vi "Auto.vi"() -> ()   [LabVIEW 2017]
uses:
  Control/Saurabh/prosucer_consumer_enum.ctl
  <vilib>/Utility/error.llb/DialogType.ctl
  <vilib>/Utility/file.llb/Read Delimited Spreadsheet (string).vi
  Global/Global 1.vi
  Global/DATA LOG.vi
  <userlib>/_OpenG.lib/comparison/comparison.llb/String Changed__ogtk.vi
  <vilib>/addons/database/Connection.llb/DB Tools Open Connec (String).vi
  <vilib>/addons/database/NI_Database_API.lvlib
  <vilib>/regexp/Match Regular Expression.xnode
panel:
  out "LOG DATA":string
  out "scanner value":string
  out "PRIVIOUS DATA":string
  out "array w/ subset deleted":dbl[](array[numeric])
  out "LOG DATA 2":dbl[](array[numeric])
  out "DATA":bool
  out "Boolean 6":bool
  out "Input 3":string
  out "resulting string":string
  out "error out 5":errorcluster
  out "LOADED RECIPE":string
  out "BARCODE RECIPE 2":string(combo)
  out "match substring":string
  out "SHIFT_DATA":string[](array[string])
  out "error out 4":errorcluster
  out "length 2":i32
  out "length":i32
  out "Boolean 5":bool
  out "OP40 BARCODE STRING EMPRTY":bool
  out "OP30 BARCODE STRING EMPRTY":bool
  out "trimmed string":string
  out "Array":string[][](array[string])
  out "error out 3":errorcluster
  out "OP 61":T1 {"Cycle Time" format="%#.2g"; "Actual Flow (Lpm)" format="%#.2g"; "Pressure (Bar)" format="%#.2g"; "lt Pressure (Bar)" format="%#.2g"; "Actual Flow (ccm)" format="%#.2g"}
  out "error out":errorcluster
  out "OP 10 & OP 21":T2 {"SPRING AND SEAL PRESS CHECK LOAD(N)" format="%#.2g"; "CYCLE TIME" format="%#.2g"; "SPRING AND SEAL PRESS LOAD(N)" format="%#.2g"; "SPRING LOAD AT 13.4 mm(N)" format="%#.2g"; "SPRING LOAD AT 14 mm((N)" format="%#.2g"; "SPRING HEIGHT(mm)" format="%#.2g"; "SEAL PRESS LOAD(N)" format="%#.2g"}
  out "PLC COM.":bool
  out "STATION-4 2":T3 {"PARAMETER 10" format="%#.2g"; "PARAMETER 6" format="%#.2g"; "PARAMETER 7" format="%#.2g"; "PARAMETER 9" format="%#.2g"; "PARAMETER 8" format="%#.2g"; "CYCLE TIME" format="%#.2g"; "PARAMETER 5" format="%#.2g"; "PARAMETER 1" format="%#.2g"; "PARAMETER 2" format="%#.2g"; "PARAMETER 4" format="%#.2g"; "PARAMETER 3" format="%#.2g"}
  out "STATION-3 2":T3 {"PARAMETER 10" format="%#.2g"; "PARAMETER 6" format="%#.2g"; "PARAMETER 7" format="%#.2g"; "PARAMETER 9" format="%#.2g"; "PARAMETER 8" format="%#.2g"; "CYCLE TIME" format="%#.2g"; "PARAMETER 5" format="%#.2g"; "PARAMETER 1" format="%#.2g"; "PARAMETER 2" format="%#.2g"; "PARAMETER 4" format="%#.2g"; "PARAMETER 3" format="%#.2g"}
  out "STATION-2 2":T3 {"PARAMETER 10" format="%#.2g"; "PARAMETER 6" format="%#.2g"; "PARAMETER 7" format="%#.2g"; "PARAMETER 9" format="%#.2g"; "PARAMETER 8" format="%#.2g"; "CYCLE TIME" format="%#.2g"; "PARAMETER 5" format="%#.2g"; "PARAMETER 1" format="%#.2g"; "PARAMETER 2" format="%#.2g"; "PARAMETER 4" format="%#.2g"; "PARAMETER 3" format="%#.2g"}
  out "STATION-1 2":T4 {"PARAMETER 10" format="%#.2g"; "PARAMETER 6" format="%#.2g"; "PARAMETER 7" format="%#.2g"; "PARAMETER 9" format="%#.2g"; "PARAMETR 8" format="%#.2g"; "CYCLE TIME" format="%#.2g"; "PARAMETER 5" format="%#.2g"; "PARAMETER 1" format="%#.2g"; "PARAMETER 2" format="%#.2g"; "PARAMETER 4" format="%#.2g"; "PARAMETER 3" format="%#.2g"}
  out "stop":bool
  out "error out 2":errorcluster
  out "Shift 4":i32
  out "Time Stamp Out":timestamp[](array[timestamp]) format="%<%X>T"
  out "Time Stamp Out 4":timestamp[](array[timestamp]) format="%<%X>T"
  out "Shift_change":bool
  out "appended array":string[][](array[string])
  out "SHIFT_DATA 2":string[](array[string])
  out "SHIFT":string
  in  "error in (no error)":errorcluster
  in  "Tab Control":enum32{"Page 1", "Page 2"}(tab)
  in  "NEXT":bool
  in  "stop 2":bool
  out "Boolean":bool
  out "Boolean 2":bool
  out "Boolean 3":bool
  out "Boolean 4":bool
  out "OP 30":T5 {"Cycle Time" format="%#_2g"; "Force (KgF)" format="%#.2g"}
  out "OP 10 & OP 20":T6 {"Spring & Seal Press Check Load(N)" format="%#.2g"; "Cycle Time" format="%#.2g"; "Spring and Seal Press Load(N)" format="%#.2g"; "Load at 13.4 mm(N)" format="%#.2g"; "Load at 14 mm(N)" format="%#.2g"; "Spring Height (mm)" format="%#.2g"; "Seal Press Load (N)" format="%#.2g"}
  out "OP 40":T7 {"Calibration Pressure (Bar)" format="%#.2g"; "Fixing Ring Displacement (mm)" format="%#.2g"; "Cycle Time" format="%#.2g"; "Calibration Flow Rate (Lph)" format="%#.2g"; "Flushing Flow (Lph)" format="%#.2g"; "Flushing Pressure (Bar)" format="%#.2g"; "Calibration Displacement (mm)" format="%#.2g"; "Calibration Load (KgF)" format="%#.2g"}
  out "OP 60":T8 {"Cycle Time" format="%#.2g"; "Actual Flow (Lpm)" format="%#.2g"; "Pressure (Bar)" format="%#.2g"; "Pressure (Bar)" format="%#.2g"; "Actual Flow (ccm)" format="%#.2g"}
  in  "Add Button":bool
  in  "BARCODE RECIPE":string(combo)
  in  "Back":bool
  # "STATION 2 VALVE OPENING TEST"
  # "STATION 3 LEAK TEST"
  # "STATION 1 SPRING CHECKING"
  # "STATION 2 SPRING & SEAL ASSEMBLY"
  # "STATION 3 COVER & SUB ASSEMBLY"
  # "STATION 1 SPRING CHECKING"
  # "STATION 2 SPRING & SEAL ASSEMBLY"
  # "STATION 3 COVER & SUB ASSEMBLY"
  # "STATION 2 VALVE OPENING TEST"
  # "STATION 3 LEAK TEST"
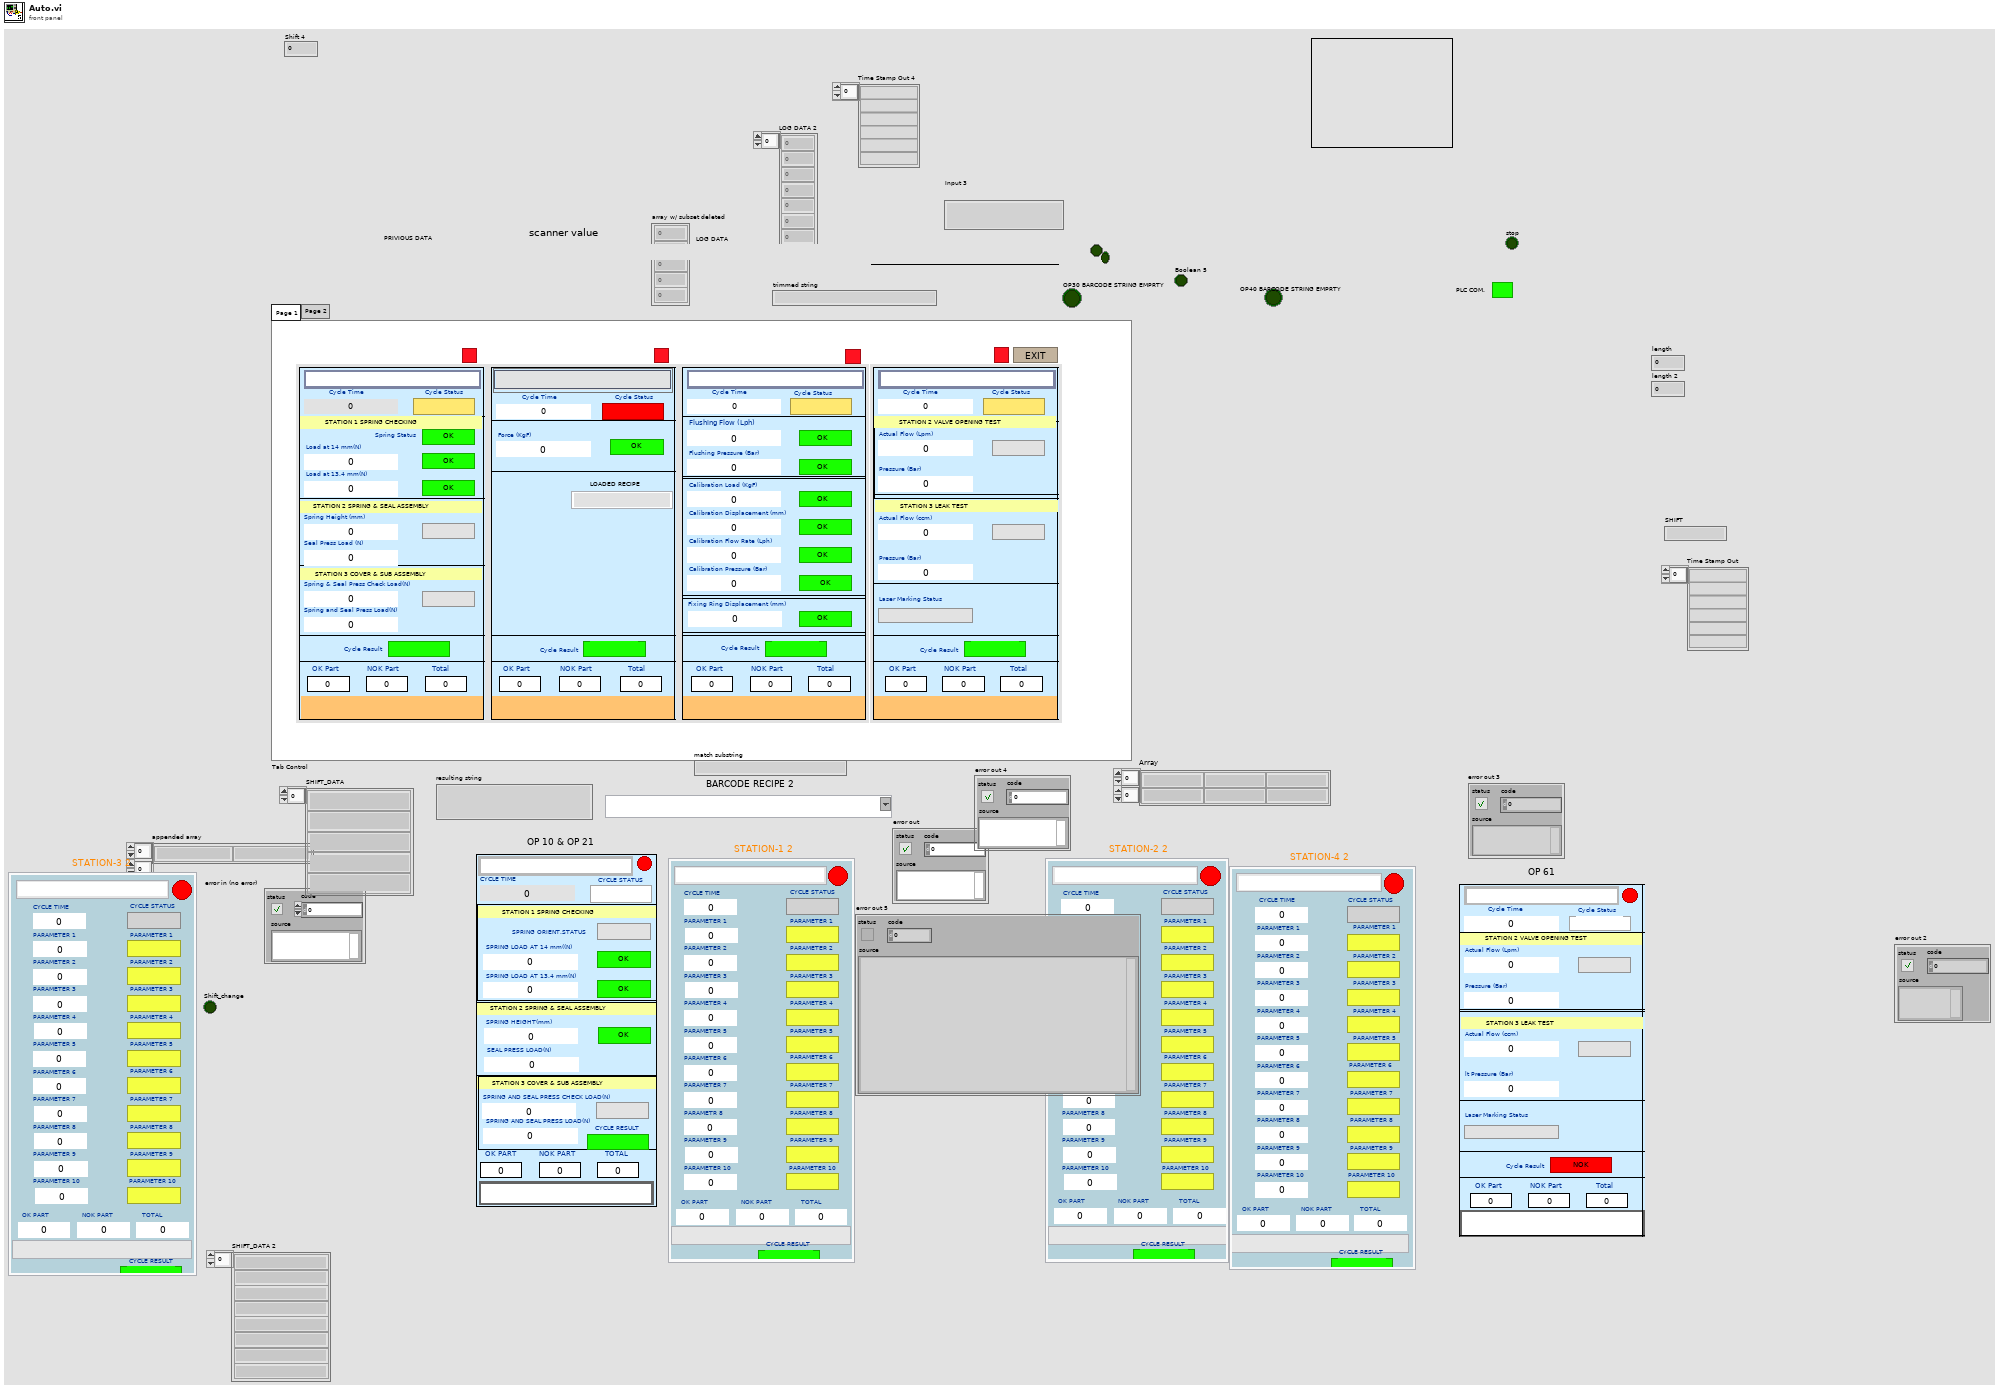
[diagram p1: front panel]
types:
  T1 = cluster{"BARCODE":string, "Cycle Time ":dbl, "Actual Flow (Lpm)":dbl, "Pressure (Bar)":dbl, "Actual Flow (ccm)":dbl, "lt Pressure (Bar)":dbl, "PARAMETER 5":dbl, "PARAMETER 6":dbl, "PARAMETER 7":dbl, "PARAMETER 8":dbl, "PARAMETER 9":dbl, "PARAMETER 10":dbl, "STATUS":string, "SCANNER":bool, "Cycle Status":bool, "VALVE OPENING TEST ACTUAL FLOW":bool, "LEAK TEST ACTUAL FLOW":bool, "Laser Marking Status":bool, "PARAMETER 4":bool, "PARAMETER 5":bool, "PARAMETER 6":bool, "PARAMETER 7":bool, "PARAMETER 8":bool, "PARAMETER 9":bool, "PARAMETER 10":bool, "OK Part":dbl, "NOK Part":dbl, "Total ":dbl, "Cycle Result":bool}
  T2 = cluster{"BARCODE":string, "CYCLE TIME":dbl, "SPRING LOAD AT 13.4 mm(N)":dbl, "SPRING LOAD AT 14 mm((N)":dbl, "SEAL PRESS LOAD(N)":dbl, "SPRING HEIGHT(mm)":dbl, "SPRING AND SEAL PRESS LOAD(N)":dbl, "SPRING AND SEAL PRESS CHECK LOAD(N)":dbl, "PARAMETER 7":dbl, "PARAMETR 8":dbl, "PARAMETER 9":dbl, "PARAMETER 10":dbl, "STATUS":string, "SCANNER":bool, "CYCLE STATUS":bool, "SPRING ORIENT.STATUS":bool, "SPRING LOAD AT 13.4 mm":bool, "SPRING LOAD AT 14 mm":bool, "SEAL PRESS LOAD(N)":bool, "SPRING HEIGHT(mm)":bool, "SPRING AND SEAL PRESS LOAD(N)":bool, "SPRING AND SEAL PRESS CHECK LOAD(N)":bool, "PARAMETER 8":bool, "PARAMETER 9":bool, "PARAMETER 10":bool, "OK PART":dbl, "NOK PART":dbl, "TOTAL ":dbl, "CYCLE RESULT":bool}
  T3 = cluster{"BARCODE":string, "CYCLE TIME":dbl, "PARAMETER 1":dbl, "PARAMETER 2":dbl, "PARAMETER 3":dbl, "PARAMETER 4":dbl, "PARAMETER 5":dbl, "PARAMETER 6":dbl, "PARAMETER 7":dbl, "PARAMETER 8":dbl, "PARAMETER 9":dbl, "PARAMETER 10":dbl, "STATUS":string, "SCANNER":bool, "CYCLE STATUS":bool, "PARAMETER 1":bool, "PARAMETER 2":bool, "PARAMETER 3":bool, "PARAMETER 4":bool, "PARAMETER 5":bool, "PARAMETER 6":bool, "PARAMETER 7":bool, "PARAMETER 8":bool, "PARAMETER 9":bool, "PARAMETER 10":bool, "OK PART":dbl, "NOK PART":dbl, "TOTAL ":dbl, "CYCLE RESULT":bool}
  T4 = cluster{"BARCODE":string, "CYCLE TIME":dbl, "PARAMETER 1":dbl, "PARAMETER 2":dbl, "PARAMETER 3":dbl, "PARAMETER 4":dbl, "PARAMETER 5":dbl, "PARAMETER 6":dbl, "PARAMETER 7":dbl, "PARAMETR 8":dbl, "PARAMETER 9":dbl, "PARAMETER 10":dbl, "STATUS":string, "SCANNER":bool, "CYCLE STATUS":bool, "PARAMETER 1":bool, "PARAMETER 2":bool, "PARAMETER 3":bool, "PARAMETER 4":bool, "PARAMETER 5":bool, "PARAMETER 6":bool, "PARAMETER 7":bool, "PARAMETER 8":bool, "PARAMETER 9":bool, "PARAMETER 10":bool, "OK PART":dbl, "NOK PART":dbl, "TOTAL ":dbl, "CYCLE RESULT":bool}
  T5 = cluster{"BARCODE":string, "Cycle Time":dbl, "Force (KgF)":dbl, "POSITION (mm)":dbl, "PARAMETER 3":dbl, "PARAMETER 4":dbl, "PARAMETER 5":dbl, "PARAMETER 6":dbl, "PARAMETER 7":dbl, "PARAMETER 8":dbl, "PARAMETER 9":dbl, "PARAMETER 10":dbl, "STATUS":string, "SCANNER":bool, "Cycle Status":bool, "FORCE (N)":bool, "POSITION (mm)":bool, "PARAMETER 3":bool, "PARAMETER 4":bool, "PARAMETER 5":bool, "PARAMETER 6":bool, "PARAMETER 7":bool, "PARAMETER 8":bool, "PARAMETER 9":bool, "PARAMETER 10":bool, "OK Part":dbl, "NOK Part":dbl, "Total ":dbl, "Cycle Result":bool}
  T6 = cluster{"BARCODE":string, "Cycle Time":dbl, " Load at 13.4 mm(N)":dbl, " Load at 14 mm(N)":dbl, "Seal Press Load (N)":dbl, "Spring Height (mm)":dbl, "Spring and Seal Press Load(N)":dbl, "Spring & Seal Press Check Load(N)":dbl, "PARAMETER 7":dbl, "PARAMETR 8":dbl, "PARAMETER 9":dbl, "PARAMETER 10":dbl, "STATUS":string, "SCANNER":bool, "Cycle Status":bool, "Spring Status":bool, "SPRING LOAD AT 13.4 mm":bool, "SPRING LOAD AT 14 mm":bool, "SEAL PRESS LOAD(N)":bool, "SPRING HEIGHT(mm)":bool, "SPRING AND SEAL PRESS LOAD(N)":bool, "SPRING AND SEAL PRESS CHECK LOAD(N)":bool, "PARAMETER 8":bool, "PARAMETER 9":bool, "PARAMETER 10":bool, "OK Part":dbl, "NOK Part":dbl, "Total ":dbl, "Cycle Result":bool}
  T7 = cluster{"BARCODE":string, "Cycle Time":dbl, "Flushing Flow (Lph)":dbl, "Flushing Pressure (Bar)":dbl, "Calibration Load (KgF) ":dbl, "Calibration Displacement (mm) ":dbl, "Calibration Flow Rate (Lph)":dbl, "Calibration Pressure (Bar)":dbl, "Fixing Ring Displacement (mm)":dbl, "PARAMETER 8":dbl, "PARAMETER 9":dbl, "PARAMETER 10":dbl, "STATUS":string, "SCANNER":bool, "Cycle Status":bool, "FLUSHING FLOW RATE":bool, "FLUSHING PRESSURE":bool, "CALIBRATION LOAD VALUE":bool, "CALIBRATION DISPLACEMENT VALUE":bool, "CALIBRATION FLOW RATE":bool, "CALIBRATION PRESSURE":bool, "FIXING RING DISPLACEMENT":bool, "PARAMETER 8":bool, "PARAMETER 9":bool, "PARAMETER 10":bool, "OK Part":dbl, "NOK Part":dbl, "Total ":dbl, "Cycle Result":bool}
  T8 = cluster{"BARCODE":string, "Cycle Time ":dbl, "Actual Flow (Lpm)":dbl, "Pressure (Bar)":dbl, "Actual Flow (ccm)":dbl, "Pressure (Bar)":dbl, "PARAMETER 5":dbl, "PARAMETER 6":dbl, "PARAMETER 7":dbl, "PARAMETER 8":dbl, "PARAMETER 9":dbl, "PARAMETER 10":dbl, "STATUS":string, "SCANNER":bool, "Cycle Status":bool, "VALVE OPENING TEST ACTUAL FLOW":bool, "LEAK TEST ACTUAL FLOW":bool, "Laser Marking Status":bool, "PARAMETER 4":bool, "PARAMETER 5":bool, "PARAMETER 6":bool, "PARAMETER 7":bool, "PARAMETER 8":bool, "PARAMETER 9":bool, "PARAMETER 10":bool, "OK Part":dbl, "NOK Part":dbl, "Total ":dbl, "Cycle Result":bool}
  T9 = typedef "prosucer_consumer_enum.ctl" = enum16{"SCAN1", "SCAN2", "SCAN3", "SCAN4", "STOP", "DATALOG1", "DATALOG2", "DATALOG3", "DATALOG4", "-1", "CYCLE_START1", "CYCLE_START2", "CYCLE_START3", "CYCLE_START4", "BARCODE RECIPE", "EMERGENCY STOP"}
  T10 = enum32{"invalid app kind", "Development System", "Run Time System", "Student Edition", "Embedded LabVIEW", "Evaluation", "Custom"}
  T11 = typedef "NI_Database_API.lvlib/Conn ObjectReference.ctl" = refnum<k1>
  T12 = typedef "DialogType.ctl" = u16
  T13 = cluster{"trimmed string":string, "SHIFT":string, "date/time string":string, dbl[], bool[], string}
  T14 = cluster{"SHIFT":string, "date/time string":string, dbl[], bool[], "CYCLE RESULT":bool, string}
  T15 = cluster{"SHIFT":string, "date/time string":string, dbl[], bool[], string}
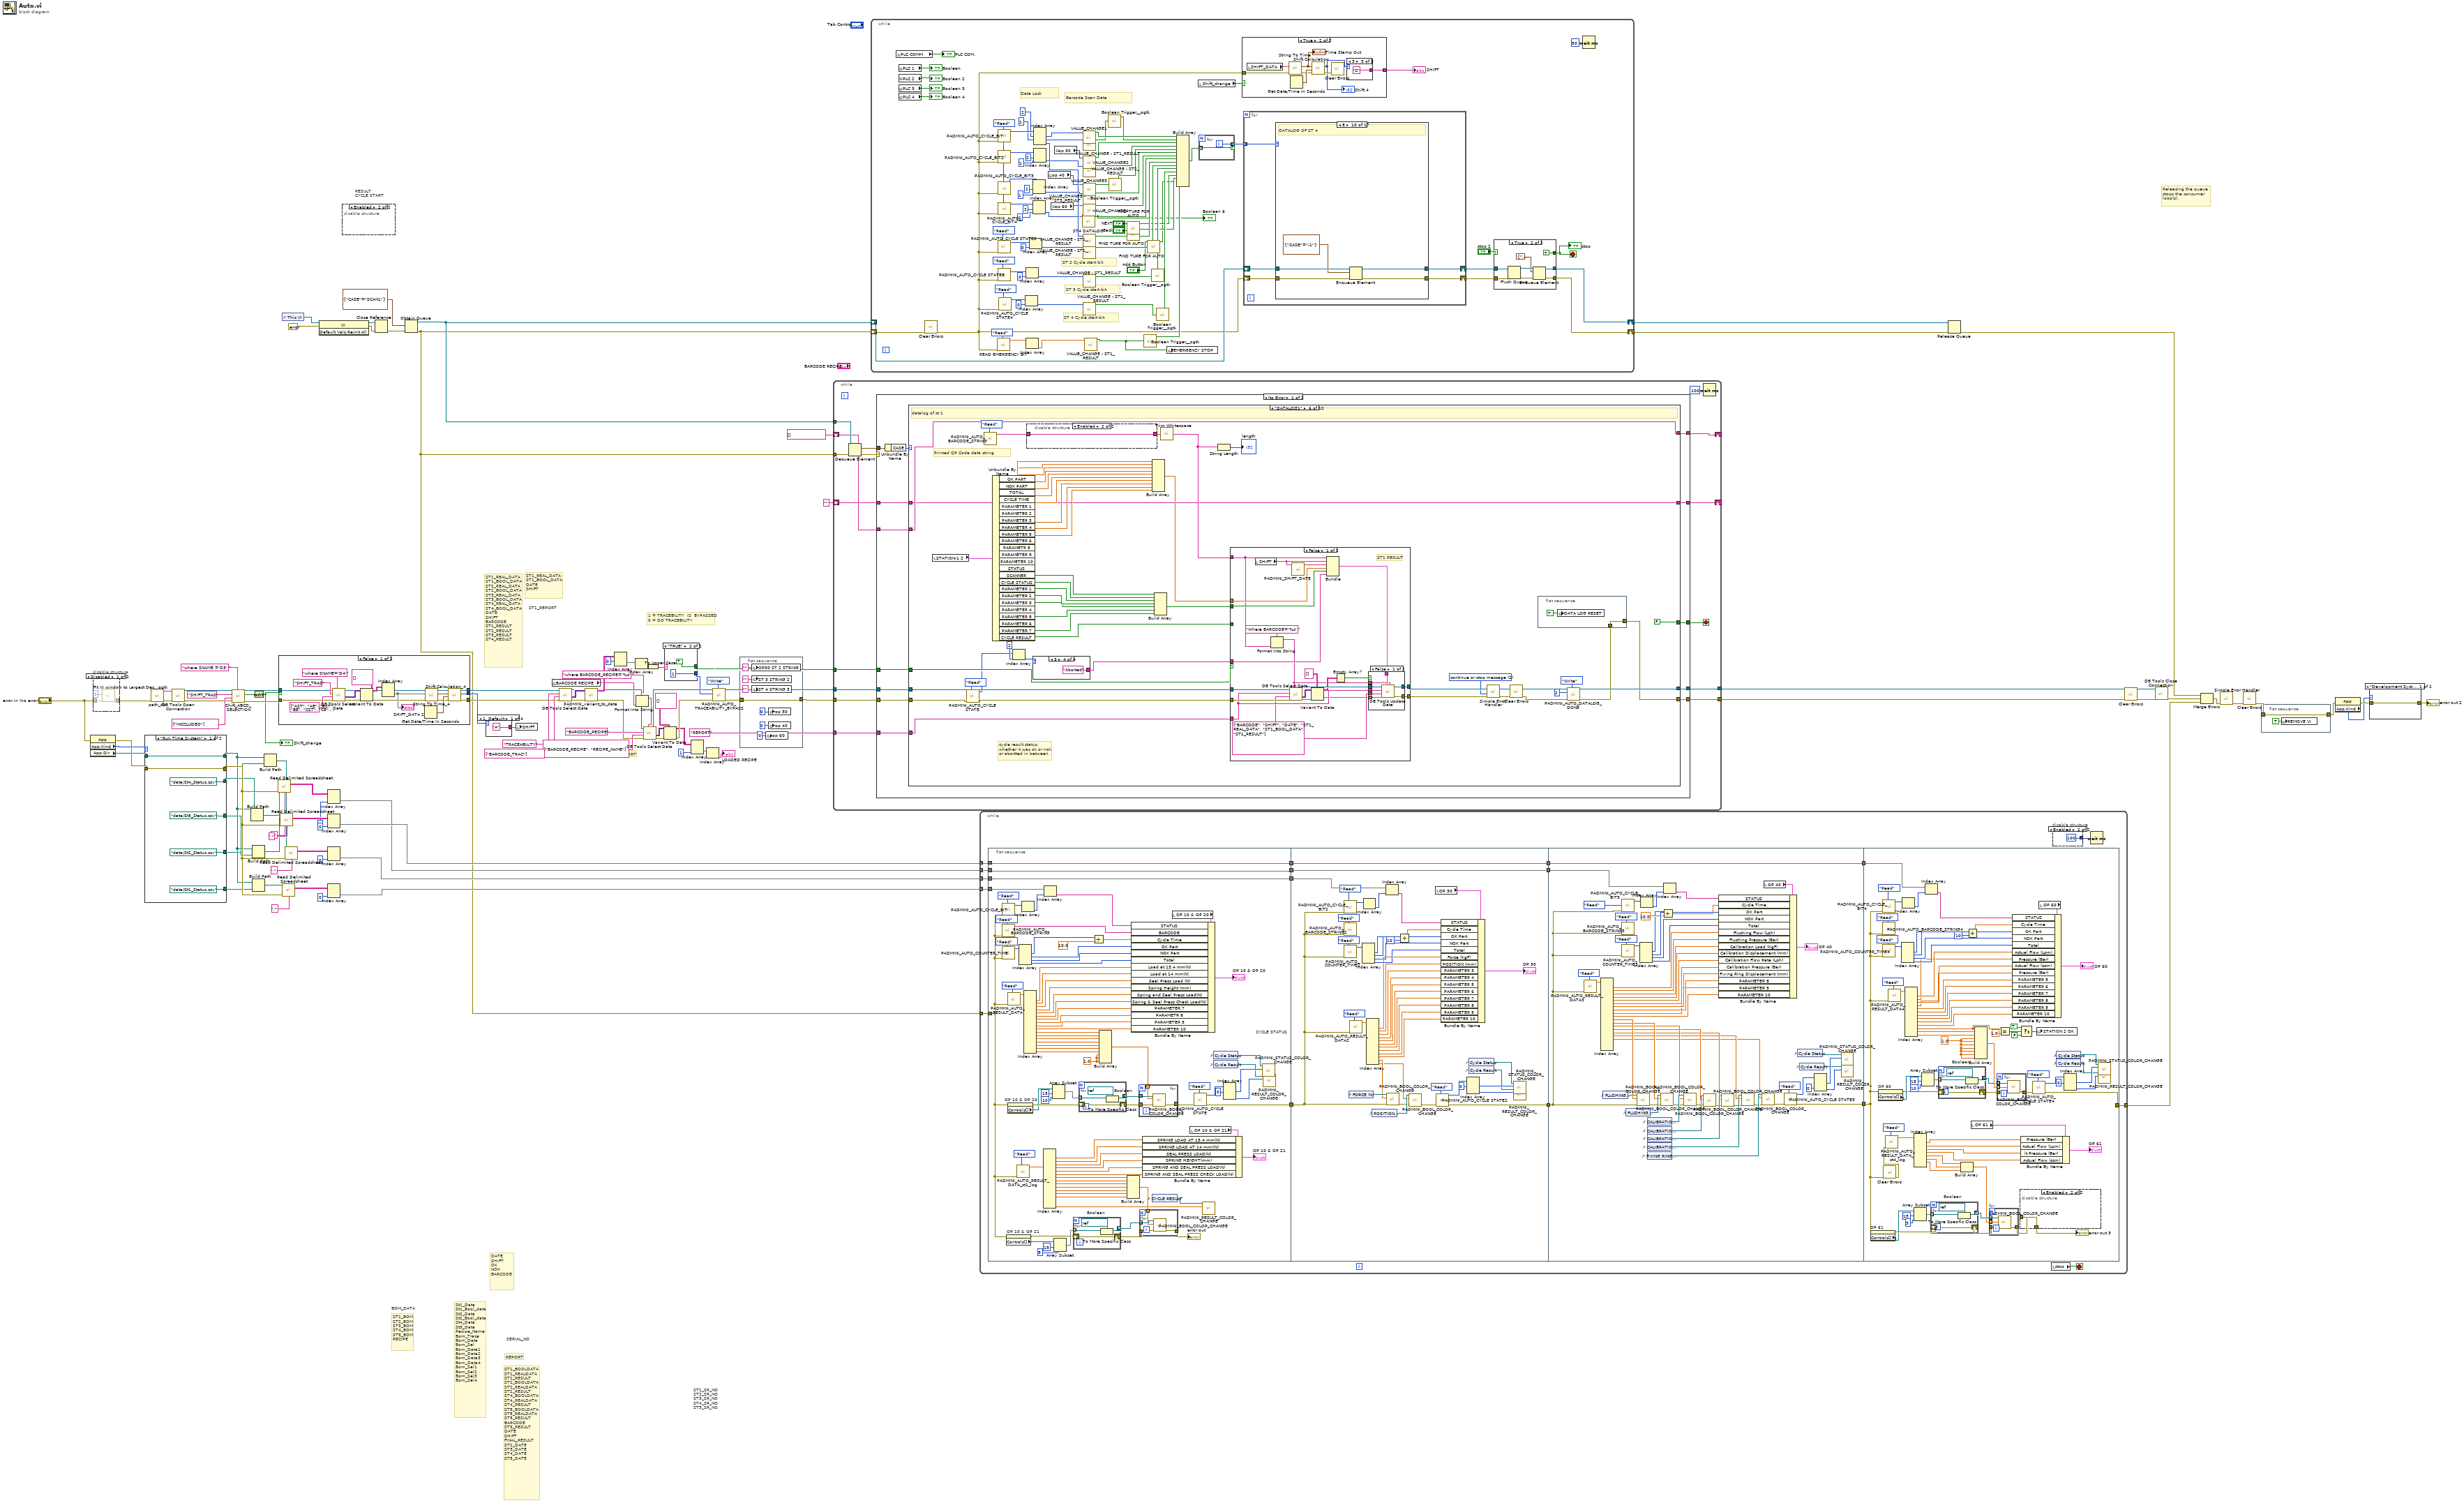
[diagram p0: block diagram]
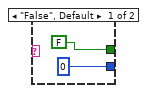
[diagram p3: hidden frame]
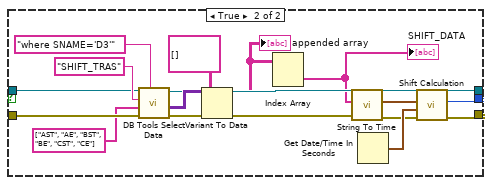
[diagram p4: hidden frame]
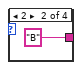
[diagram p5: hidden frame]
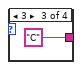
[diagram p6: hidden frame]
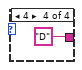
[diagram p7: hidden frame]
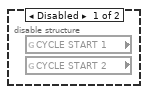
[diagram p8: hidden frame]
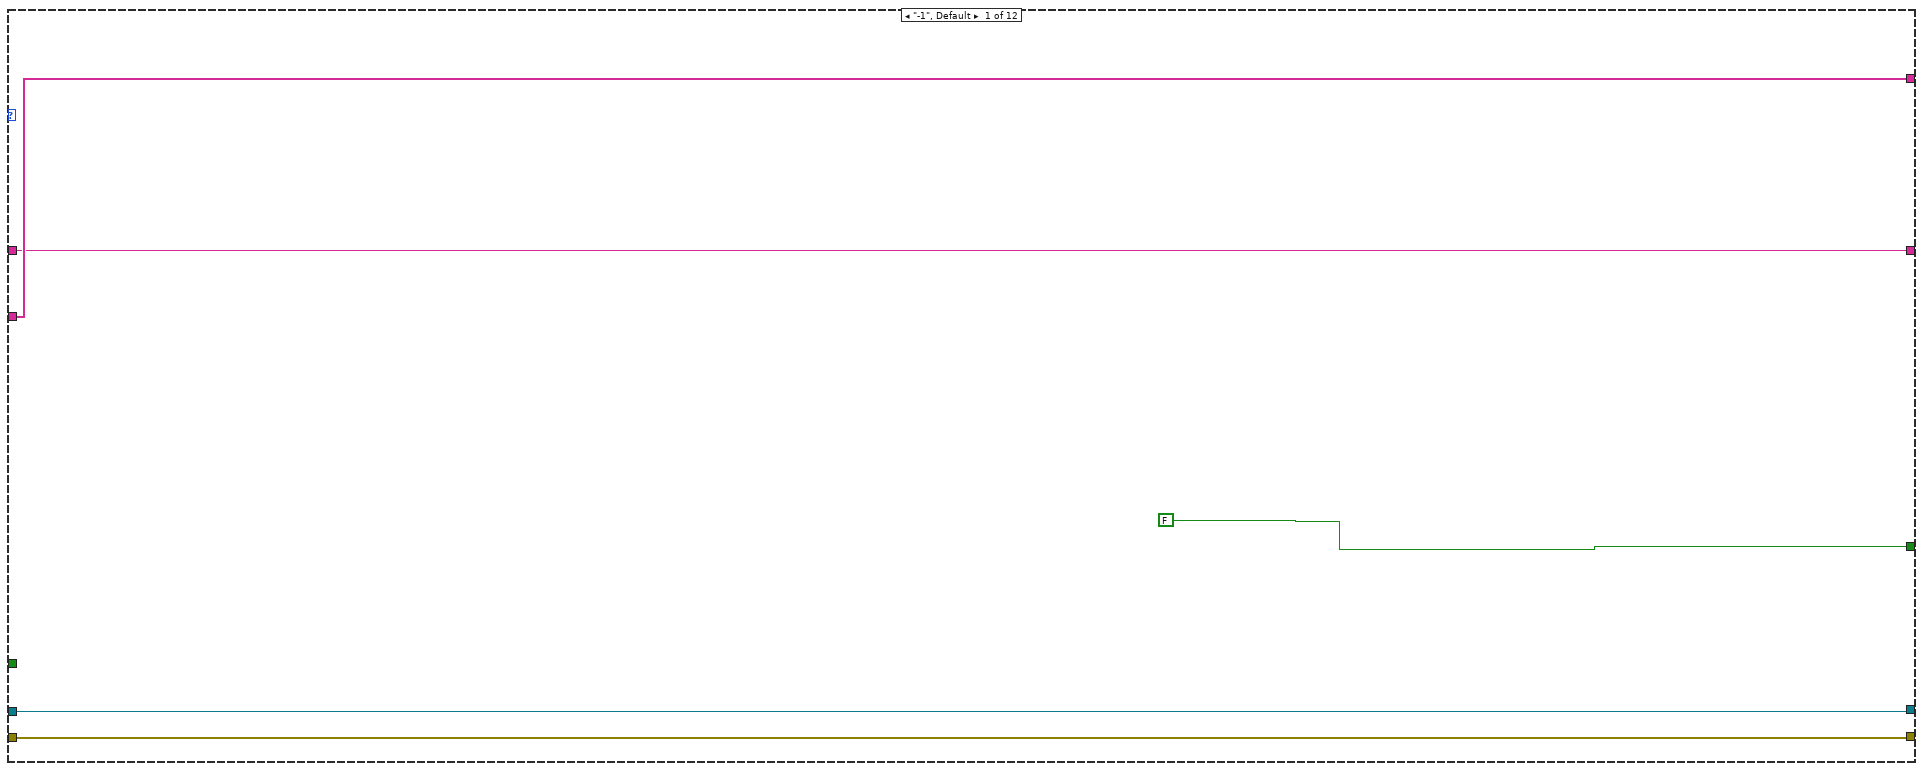
[diagram p9: hidden frame]
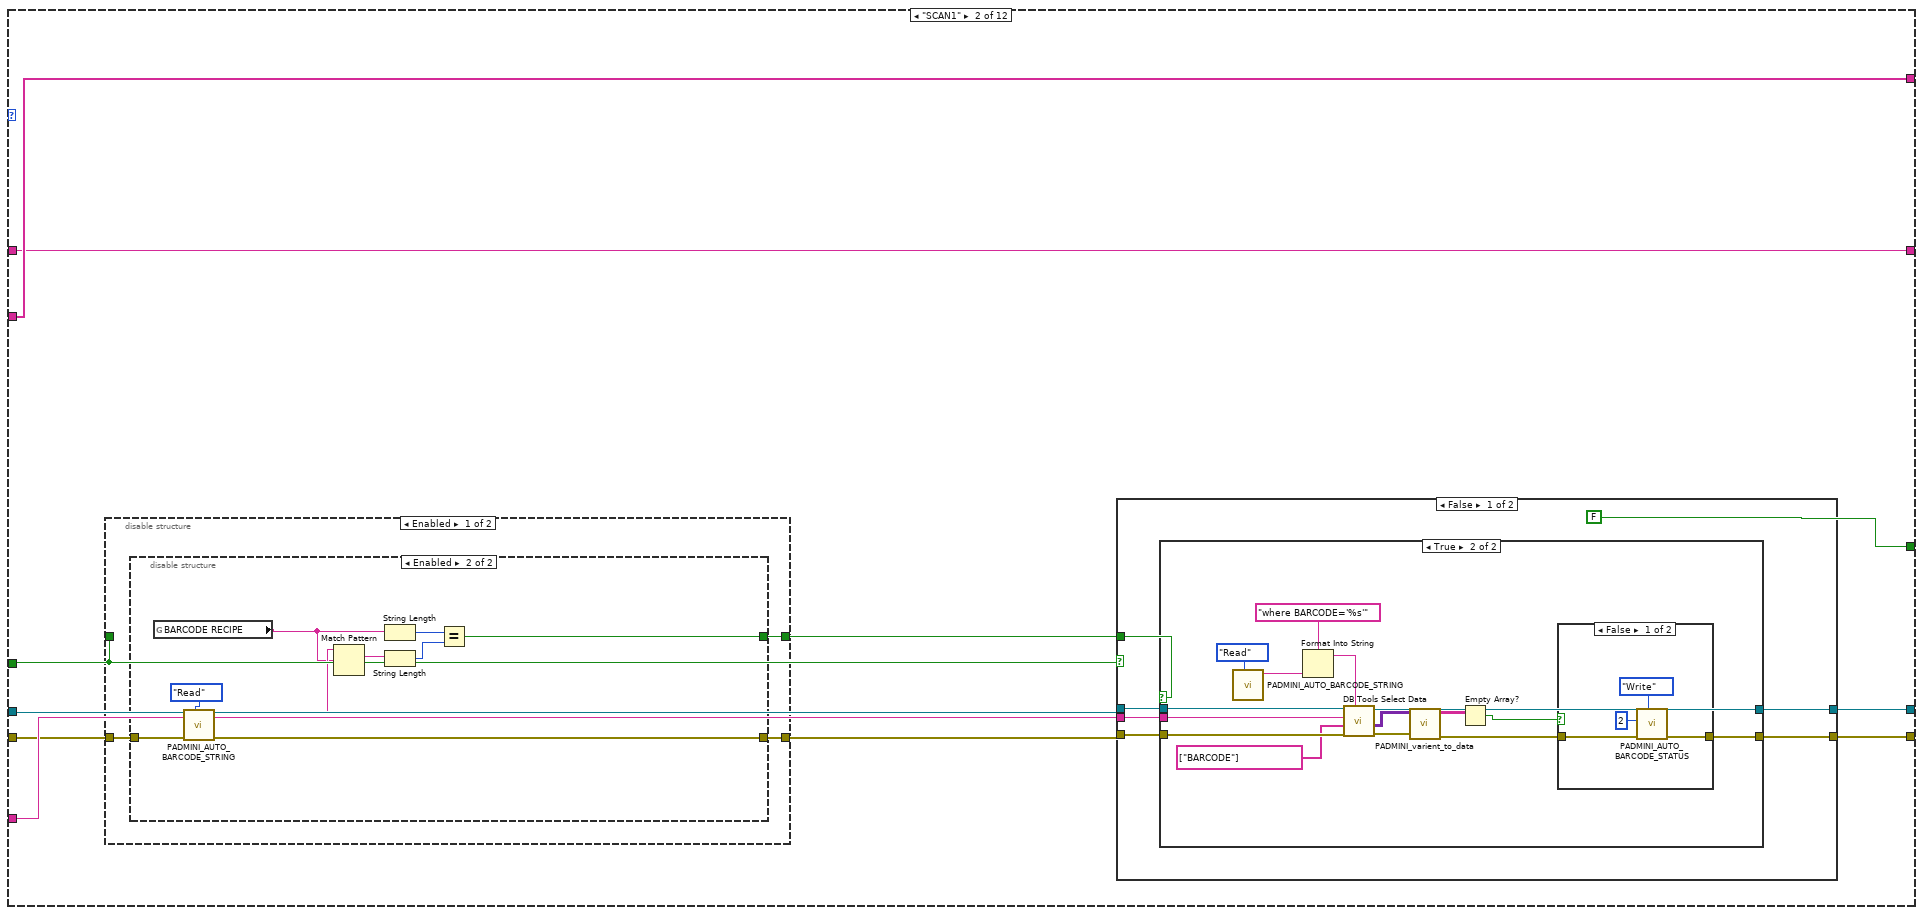
[diagram p10: hidden frame]
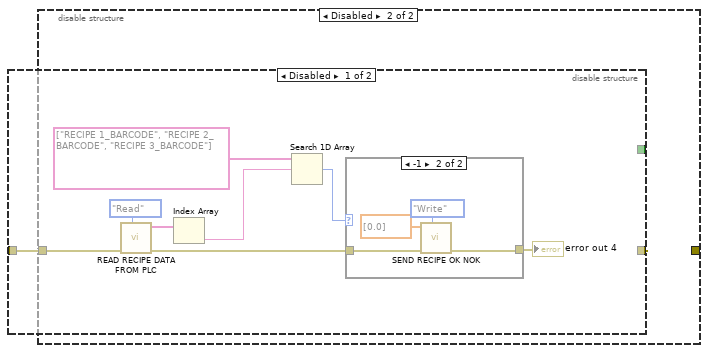
[diagram p11: hidden frame]
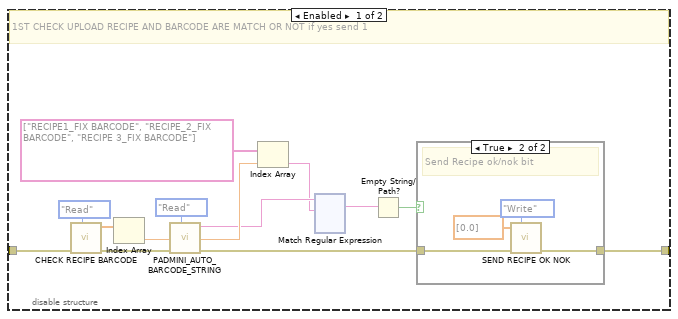
[diagram p12: hidden frame]
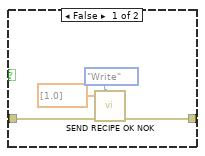
[diagram p13: hidden frame]
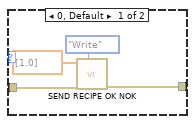
[diagram p14: hidden frame]
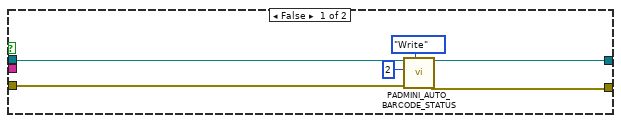
[diagram p16: hidden frame]
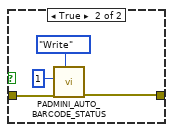
[diagram p17: hidden frame]
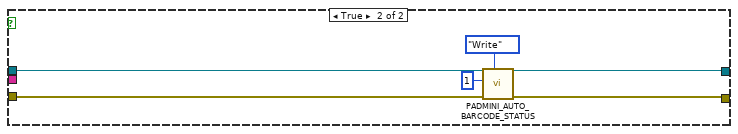
[diagram p18: hidden frame]
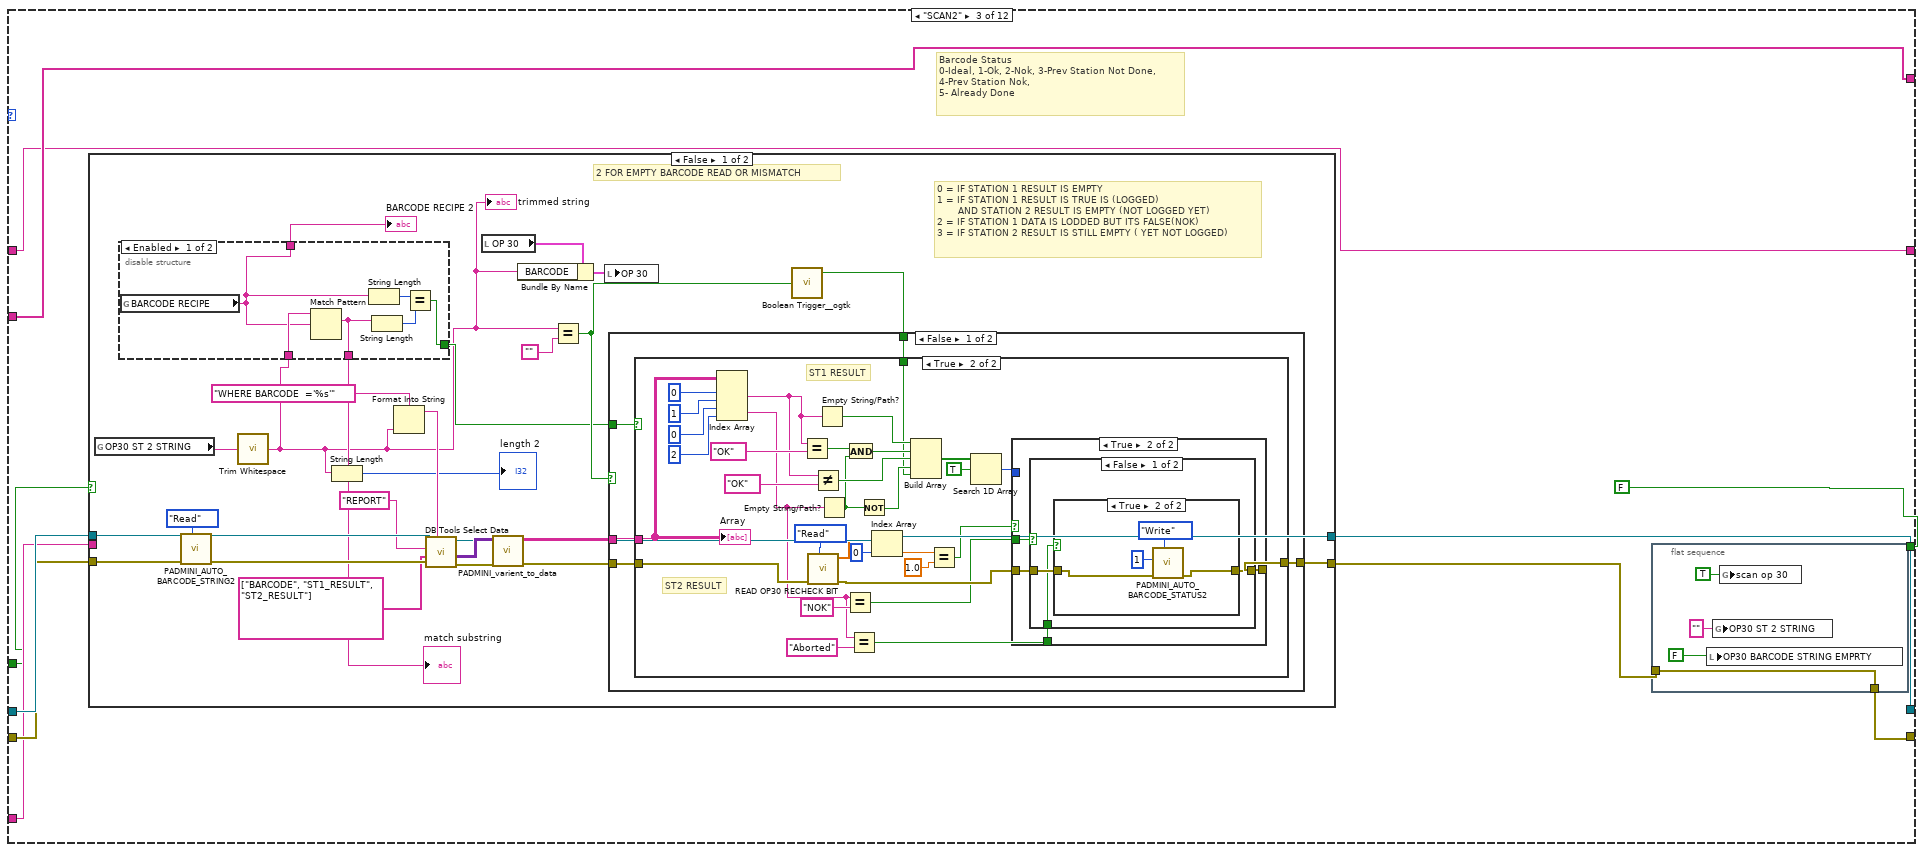
[diagram p19: hidden frame]
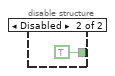
[diagram p20: hidden frame]
diagram:
  # "1 = TRACEBILITY  IS  BYPASSED\n0 = DO TRACEBILITY"
  # "ST1_REAL_DATA\nST1_BOOL_DATA\nST2_REAL_DATA\nST2_BOOL_DATA\nST3_REAL_DATA\nST3_BOOL_DATA\nST4_REAL_DATA\nST4_BOOL_DATA\nDATE\nSHIFT\nBARCODE\nST1_RESULT\nST2_RESULT\nST3_RESULT\nST4_RESULT"
  # "ST1_REPORT"
  # "ST1_REAL_DATA\nST1_BOOL_DATA\nDATE\nSHIFT"
  # "REPORT"
  # "DATE\nSHIFT\nOK\nNOK\nBARCODE"
  # "REPORT"
  # "ST1_BOOLDATA\nST1_REALDATA\nST1_RESULT\nST2_BOOLDATA\nST2_REALDATA\nST2_RESULT\nST4_BOOLDATA\nST4_REALDATA\nST4_RESULT\nST5_BOOLDATA\nST5_REALDATA\nST5_RESULT\nBARCODE\nST3_RESULT\nDATE\nSHIFT\nFINAL_RESULT\nST2_DATE\nST3_DATE\nST4_DATE\nST5_DATE"
  # "SERIAL_NO"
  # "ST1_SR_NO\nST2_SR_NO\nST3_SR_NO\nST4_SR_NO\nST5_SR_NO"
  # "RESULT\nCYCLE START"
  # "St1_Data\nSt1_Bool_data\nSt2_Data\nSt2_Bool_data\nSt4_Data\nSt5_Data\nRecipe_Name\nBom_Trace\nBom_Data\nBom_Sel\nBom_Data1\nBom_Data2\nBom_Data3\nBom_Data4\nBom_Sel1\nBom_Sel2\nBom_Sel3\nBom_Sel4"
  # "BOM_DATA"
  # "ST1_BOM\nST2_BOM\nST3_BOM\nST4_BOM\nST5_BOM\nRECIPE"
  # "Releasing the queue stops the consumer loop(s)."
  n1 = property class="App"(error in="error in (no error)") -> (error out=w84:errorcluster, "App.Kind"=w86:T10, "App.Dir"=w85:path)  [unwired: 1 in, 1 out]
  n2 = disable-structure shown="Disabled" {
    disable-tunnel: "error in (no error)" -> [w105 w106]
    disable-tunnel: [w104 w106] -> w37
    frame Disabled {
      n3 = call <userlib>:"Fit VI window to Largest Dec__ogtk.vi"("error in (no error)"=w105, "border spacing (2 px)"=0) -> ("error out"=w104:errorcluster)  [unwired: 4 in, 1 out]
    }
    frame Enabled {
    }
  }
  n4 = case shown="\"Run Time System\"" w86 {
    tunnel: w85 -> [w112 _]
    tunnel: [w112 w118] -> w49
    tunnel: w84 -> [w111 w117]
    tunnel: [w111 w117] -> w50
    tunnel: [path "data/St4_Status.csv" ("path") path "../data/St4_Status.csv" ("path")] -> w48
    tunnel: [path "data/St3_Status.csv" ("path") path "../data/St3_Status.csv" ("path")] -> w47
    tunnel: [path "data/St2_Status.csv" ("path") path "../data/St2_Status.csv" ("path")] -> w46
    tunnel: [path "data/St1_Status.csv" ("path") path "../data/St1_Status.csv" ("path")] -> w45
    frame "Run Time System" {
    }
    frame Default {
      n5 = Current VI's Path() -> (path=w119:path)
      n6 = Strip Path(path=w119) -> (stripped path=w118:path)  [unwired: 1 out]
    }
  }
  n7 = call "path_db.vi"("error in"=w37) -> ("error out"=w74:errorcluster, "resulting string"=w99:string)  [unwired: 9 in]
  n8 = call-poly <vilib>:"DB Tools Open Connection.vi"("error in (no error)"=w74, "connection information"=w99) -> ("error out"=w73:errorcluster, "connection reference"=w43:T11)  [unwired: 6 in]
  n9 = call "Shift_ABCD_SELECTION.vi"("Where"="where SNAME ='D3' ", "error in (no error)"=w73, "Array"=string[] ["INCCLUDED"], "table"="SHIFT_TRAS", "Refnum in"=w43) -> ("error out"=w90:errorcluster, "Boolean"=w89:bool, "Refnum out"=w91:T11)  [unwired: 4 in]
  n10 = Build Path(base path=w49, name or relative path=w48) -> (appended path=w64:path)
  n11 = Build Path(base path=w49, name or relative path=w47) -> (appended path=w61:path)
  n12 = Build Path(base path=w49, name or relative path=w45) -> (appended path=w53:path)
  n13 = Not(x=w89) -> (.not. x?=w88:bool)
  "Shift_change" <- w88
  n14 = Build Path(base path=w49, name or relative path=w46) -> (appended path=w56:path)
  n15 = call-poly <vilib>:"Read Delimited Spreadsheet.vi"("file path (dialog if empty)"=w61, "error in (no error)"=w50, "delimiter (\\t)"="," ("delimiter (\\t)")) -> ("all rows"=w60:string[][])  [unwired: 7 in, 5 out]
  n16 = case shown="False" w88 {
    tunnel: [w121 w145] -> w95
    tunnel: w91 -> [w124 w143]
    tunnel: w90 -> [w123 w142]
    tunnel: [w122 w141] -> w27
    tunnel: [w120 w135] -> w26
    frame False {
      n17 = call <vilib>:"DB Tools Select Data.vi"("condition"="where SNAME='D4'", "error in (no error)"=w123, "columns"=string[] ["AST", "AE", "BST", "BE", "CST", "CE", "DST", "DE"], "table"="SHIFT_TRAS", "connection reference"=w124) -> ("error out"=w130:errorcluster, "data"=w134:variant[][], "connection reference out"=w122:T11)  [unwired: 1 in]
      n18 = Variant To Data(error in=w130, type=string[][] [], Variant=w134) -> (data=w127:string[][], error out=w120:errorcluster)
      n19 = Index Array(array=w127) -> (element=w126:string[])  [unwired: 2 in]
      "SHIFT_DATA 2" <- w126
      n20 = Get Date/Time In Seconds() -> (seconds since 1Jan1904=w129:timestamp)
      n21 = call "String To Time_4.vi"("String Array In"=w126) -> ("Time Stamp Out"=w125:timestamp[])  [unwired: 9 in, 1 out]
      n22 = call "Shift Calculation_4.vi"("Current Time"=w129, "Time Stamp Out"=w125) -> ("Shift"=w121:i32)  [unwired: 8 in, 1 out]
    }
    frame True {
      n23 = call <vilib>:"DB Tools Select Data.vi"("condition"="where SNAME='D3'", "error in (no error)"=w142, "columns"=string[] ["AST", "AE", "BST", "BE", "CST", "CE"], "table"="SHIFT_TRAS", "connection reference"=w143) -> ("error out"=w147:errorcluster, "data"=w151:variant[][], "connection reference out"=w141:T11)  [unwired: 1 in]
      n24 = Variant To Data(error in=w147, type=string[][] [], Variant=w151) -> (data=w139:string[][], error out=w137:errorcluster)
      "appended array" <- w139
      n25 = Index Array(array=w139) -> (element=w138:string[])  [unwired: 2 in]
      "SHIFT_DATA" <- w138
      n26 = call "String To Time.vi"("error in (no error)"=w137, "String Array In"=w138) -> ("error out"=w136:errorcluster, "Time Stamp Out"=w144:timestamp[])  [unwired: 8 in]
      n27 = Get Date/Time In Seconds() -> (seconds since 1Jan1904=w146:timestamp)
      n28 = call "Shift Calculation.vi"("error in (no error)"=w136, "Current Time"=w146, "Time Stamp Out"=w144) -> ("error out"=w135:errorcluster, "Shift"=w145:i32)  [unwired: 7 in]
    }
  }
  n29 = call-poly <vilib>:"Read Delimited Spreadsheet.vi"("file path (dialog if empty)"=w64, "error in (no error)"=w50, "delimiter (\\t)"="," ("delimiter (\\t)")) -> ("all rows"=w65:string[][])  [unwired: 7 in, 5 out]
  n30 = control-ref of="This VI"() -> (w71:refnum<vi>)
  n31 = call-poly <vilib>:"Read Delimited Spreadsheet.vi"("file path (dialog if empty)"=w53, "error in (no error)"=w50, "delimiter (\\t)"="," ("delimiter (\\t)")) -> ("all rows"=w52:string[][])  [unwired: 7 in, 5 out]
  n32 = call-poly <vilib>:"Read Delimited Spreadsheet.vi"("file path (dialog if empty)"=w56, "error in (no error)"=w50, "delimiter (\\t)"="," ("delimiter (\\t)")) -> ("all rows"=w57:string[][])  [unwired: 7 in, 5 out]
  n33 = invoke class="VI" method="Default Vals.Reinit All"(reference=w71, error in=errorcluster {"status"=FALSE, "code"=0, "source"=""} ("error in (no error)")) -> (reference out=w69:refnum<vi>, error out=w70:errorcluster)  [unwired: 1 in, 1 out]
  n34 = Index Array(array=w60, index (col)=0 ("disabled index (col)")) -> (element=w40:string[])  [unwired: 1 in]
  n35 = Index Array(array=w65, index (col)=0 ("disabled index (col)")) -> (element=w42:string[])  [unwired: 1 in]
  n36 = Index Array(array=w57, index (col)=0 ("disabled index (col)")) -> (element=w39:string[])  [unwired: 1 in]
  n37 = Index Array(array=w52, index (col)=0 ("disabled index (col)")) -> (element=w41:string[])  [unwired: 1 in]
  n38 = disable-structure shown="Enabled" {
    frame Disabled {
      n39 = global read "Global 1.vi" "CYCLE START 1"() -> ()  [unwired: 1 out]
      n40 = global read "Global 1.vi" "CYCLE START 2"() -> ()  [unwired: 1 out]
    }
    frame Enabled {
    }
  }
  n41 = Close Reference(reference=w69, error in (no error)=w70) -> (error out=w67:errorcluster)
  n42 = Obtain Queue(element data type=cluster{"CASE":T9} {"CASE"=enum."SCAN1"}, error in (no error)=w67) -> (queue out=w100:refnum<queue>, error out=w19:errorcluster)  [unwired: 3 in, 1 out]
  n43 = case shown="1, Default" w95 {
    tunnel: ["A" "B" "C" "D"] -> w87
    frame 1, Default {
    }
    frame 2 {
    }
    frame 3 {
    }
    frame 4 {
    }
  }
  n44 = local write "SHIFT"(w87) -> ()
  n45 = global read "Global 1.vi" "BARCODE RECIPE"() -> (w7:string)
  n46 = call <vilib>:"DB Tools Select Data.vi"("error in (no error)"=w26, "columns"=string[] ["BARCODE_TRAC"], "table"="TRACEABILITY", "connection reference"=w27) -> ("error out"=w36:errorcluster, "data"=w35:variant[][], "connection reference out"=w13:T11)  [unwired: 2 in]
  n47 = call "PADMINI_varient_to_data.vi"("error in (no error)"=w36, "data"=w35) -> ("error out"=w11:errorcluster, "Array"=w34:string[][])  [unwired: 8 in]
  n48 = Index Array(array=w34, index (row)=0 ("disabled index (col)")) -> (element=w33:string[])  [unwired: 1 in]
  n49 = Index Array(array=w33) -> (element=w29:string)  [unwired: 1 in]
  n50 = Format Into String(format string="where BARCODE_RECIPE='%s' ", w7) -> (resulting string=w5:string)  [unwired: 2 in, 1 out]
  n51 = call <vilib>:"DB Tools Select Data.vi"("condition"=w5, "error in (no error)"=w11, "columns"=string[] ["BARCODE_RECIPE", "RECIPE_NAME"], "table"="BARCODE_RECIPE", "connection reference"=w13) -> ("error out"=w15:errorcluster, "data"=w14:variant[][], "connection reference out"=w12:T11)  [unwired: 1 in]
  n52 = To Upper Case(1:w29) -> (0:w28:string)
  n53 = Variant To Data(error in=w15, type=string[][] [], Variant=w14) -> (data=w8:string[][], error out=w10:errorcluster)
  n54 = case shown="\"TRUE\"" w28 {
    tunnel: [FALSE ("BARCODE TRACEABILITY") TRUE ("BARCODE TRACEABILITY")] -> w18
    tunnel: [0 1] -> w24
    frame "False", Default {
    }
    frame "TRUE" {
    }
  }
  n55 = Index Array(array=w8, index (col)=1 ("disabled index (col)")) -> (element=w3:string[])  [unwired: 1 in]
  n56 = Index Array(array=w3) -> (element=→"LOADED RECIPE":string)  [unwired: 1 in]
  n57 = call "PADMINI_AUTO_TRACEABILITY_BYPASS.vi"("Enum"=enum16{"Read", "Write"}."Write", "error in (no error)"=w10, "I/P"=w24) -> ("error out"=w22:errorcluster)  [unwired: 7 in, 1 out]
  n58 = flat-sequence {
    tunnel: w22 -> [w163]
    tunnel: [w163] -> w21
    frame #0 {
      n59 = global write "DATA LOG.vi" "OP30 ST 2 STRING"("" ("OP30 ST 2 STRING")) -> ()
      n60 = global write "DATA LOG.vi" "ST 3 STRING 2"("" ("ST 3 STRING 2")) -> ()
      n61 = global write "DATA LOG.vi" "ST 4 STRING 3"("" ("ST 4 STRING 3")) -> ()
      n62 = global write "DATA LOG.vi" "op 60"(0 ("op 30")) -> ()
      n63 = global write "DATA LOG.vi" "op 30"(0 ("op 30")) -> ()
      n64 = global write "DATA LOG.vi" "op 40"(0 ("op 30")) -> ()
    }
  }
  n65 = while {
    tunnel: w100 -> [w182]
    tunnel: w19 -> [w178]
    tunnel: w21 -> [w177]
    tunnel: w12 -> [w176]
    tunnel: [w175] -> w98
    tunnel: [w174] -> w97
    tunnel: w18 -> [w173]
    tunnel: "REPORT" -> [w172]
    shift-right: [w170] -> _
    shift-left: string[] [] -> [w171]
    shift-right: [w169] -> _
    shift-left: "" ("trimmed string") -> [w168]
    stop <- w179 stop-if-true
    n66 = Dequeue Element(queue=w182, error in (no error)=w178) -> (element=w180:cluster{"CASE":T9}, error out=w181:errorcluster)  [unwired: 1 in, 2 out]
    n67 = case shown="No Error" w181 {
      tunnel: w180 -> [w195 _]
      tunnel: [w191 TRUE] -> w179
      tunnel: w177 -> [w192 w1338]
      tunnel: w176 -> [w193 w1337]
      tunnel: [w189 w1338] -> w175
      tunnel: [w190 w1337] -> w174
      tunnel: w173 -> [w188 _]
      tunnel: w172 -> [w187 _]
      tunnel: w171 -> [w186 w1336]
      tunnel: [w185 w1336] -> w170
      tunnel: [w184 w1335] -> w169
      tunnel: w168 -> [w183 w1335]
      frame No Error {
        n68 = Unbundle By Name(w195) -> ("CASE"=w194:T9)
        n69 = case shown="\"DATALOG1\"" w194 {
          tunnel: w193 -> [w199 w210 w427 w573 w700 w909 w1014 w1086 w1169 w1308 w1323 w1330]
          tunnel: w192 -> [w198 w205 w426 w572 w699 w893 w997 w1071 w1180 w1307 w1322 w1332]
          tunnel: [FALSE FALSE FALSE FALSE FALSE FALSE FALSE FALSE FALSE FALSE FALSE TRUE] -> w191
          tunnel: [w199 w207 w424 w570 w697 w904 w1008 w1080 w1200 w1290 w1323 w1329] -> w190
          tunnel: [w198 w208 w421 w567 w695 w900 w1004 w1077 w1196 w1285 w1322 w1331] -> w189
          tunnel: w188 -> [_ w202 w423 w569 w696 w908 w1013 w1085 w1203 _ _ _]
          tunnel: w187 -> [_ w209 w425 w571 w698 w907 w1012 w1084 w1164 _ _ _]
          tunnel: w186 -> [w197 w206 w419 w566 w693 w884 w995 w1067 w1188 w1296 w1320 w1333]
          tunnel: [w197 w206 w419 w566 w692 w884 w995 w1067 w1185 w1296 w1320 w1333] -> w185
          tunnel: [w196 w201 w418 w565 w691 w879 w990 w1062 w1174 w1283 w1319 w1324] -> w184
          tunnel: w183 -> [w196 w201 w418 w565 w690 w879 w990 w1062 w1174 w1283 w1319 w1324]
          frame "-1", Default {
          }
          frame "SCAN1" {
            n70 = disable-structure shown="Enabled" {
              disable-tunnel: w205 -> [w214 w378]
              disable-tunnel: [w213 w378] -> w204
              disable-tunnel: [w212 w377] -> w203
              disable-tunnel: w202 -> [_ w377]
              frame Enabled {
                n71 = disable-structure shown="Enabled" {
                  disable-tunnel: w214 -> [w216 w375]
                  disable-tunnel: [w215 w374] -> w213
                  disable-tunnel: [_ w370] -> w212
                  frame Disabled {
                    n72 = disable-structure shown="Disabled" {
                      disable-tunnel: w216 -> [w229 w359]
                      disable-tunnel: [w217 _] -> w215
                      frame Enabled {
                        # "1ST CHECK UPLOAD RECIPE AND BARCODE ARE MATCH OR NOT if yes send 1"
                        n73 = call "CHECK RECIPE BARCODE.vi"("Enum"=enum16{"Read", "Write"}."Read", "error in (no error)"=w229) -> ("error out"=w225:errorcluster, "output"=w227:dbl[])  [unwired: 8 in]
                        n74 = Index Array(array=w227) -> (element=w223:dbl)  [unwired: 1 in]
                        n75 = call "PADMINI_AUTO_BARCODE_STRING.vi"("Enum"=enum16{"Read", "Write"}."Read", "error in (no error)"=w225) -> ("error out"=w218:errorcluster, "Input 2"=w222:string)  [unwired: 8 in]
                        n76 = Index Array(array=string[] ["RECIPE1_FIX BARCODE", "RECIPE_2_FIX BARCODE", "RECIPE 3_FIX BARCODE"], index=w223) -> (element=w221:string)
                        n77 = xnode "Match Regular Expression"("input string"=w222, "regular expression"=w221) -> ("whole match"=w220:string)  [unwired: 4 in, 4 out]
                        n78 = Empty String/Path?(string/path=w220) -> (empty?=w219:bool)
                        n79 = case shown="True" w219 {
                          tunnel: w218 -> [w231 w236]
                          tunnel: [w230 w234] -> w217
                          frame False {
                            n80 = call "SEND RECIPE OK NOK.vi"("Enum"=enum16{"Read", "Write"}."Write", "error in (no error)"=w231, "input"=dbl[] [1.0]) -> ("error out"=w230:errorcluster)  [unwired: 7 in, 1 out]
                          }
                          frame True {
                            # "Send Recipe ok/nok bit"
                            n81 = call "SEND RECIPE OK NOK.vi"("Enum"=enum16{"Read", "Write"}."Write", "error in (no error)"=w236, "input"=dbl[] [0.0]) -> ("error out"=w234:errorcluster)  [unwired: 7 in, 1 out]
                          }
                        }
                      }
                      frame Disabled {
                        # "SEND OK/NOK FOR RECIPE LOADED"
                        n82 = call "READ RECIPE DATA FROM PLC.vi"("Enum"=enum16{"Read", "Write"}."Read", "error in (no error)"=w359) -> ("error out"=w353:errorcluster, "output"=w357:string[])  [unwired: 8 in]
                        n83 = Index Array(array=w357) -> (element=w355:string)  [unwired: 1 in]
                        n84 = Search 1D Array(1D array=string[] ["RECIPE 1_BARCODE", "RECIPE 2_BARCODE", "RECIPE 3_BARCODE"], element=w355) -> (index of element=w354:i32)  [unwired: 1 in]
                        n85 = case shown="-1" w354 {
                          tunnel: w353 -> [w363 w367]
                          tunnel: [w362 w366] -> w352
                          frame 0, Default {
                            n86 = call "SEND RECIPE OK NOK.vi"("Enum"=enum16{"Read", "Write"}."Write", "error in (no error)"=w363, "input"=dbl[] [1.0]) -> ("error out"=w362:errorcluster)  [unwired: 7 in, 1 out]
                          }
                          frame -1 {
                            n87 = call "SEND RECIPE OK NOK.vi"("Enum"=enum16{"Read", "Write"}."Write", "error in (no error)"=w367, "input"=dbl[] [0.0]) -> ("error out"=w366:errorcluster)  [unwired: 7 in, 1 out]
                          }
                        }
                        "error out 4" <- w352
                      }
                    }
                  }
                  frame Enabled {
                    n88 = global read "Global 1.vi" "BARCODE RECIPE"() -> (w368:string)
                    n89 = call "PADMINI_AUTO_BARCODE_STRING.vi"("Enum"=enum16{"Read", "Write"}."Read", "error in (no error)"=w375) -> ("error out"=w374:errorcluster, "Input 2"=w369:string)  [unwired: 8 in]
                    n90 = Match Pattern(string=w369, regular expression=w368) -> (match substring=w373:string)  [unwired: 1 in, 3 out]
                    n91 = String Length(string=w368) -> (length=w372:i32)
                    n92 = String Length(string=w373) -> (length=w371:i32)
                    n93 = Equal?(x=w372, y=w371) -> (x = y?=w370:bool)
                  }
                }
              }
              frame Disabled {
              }
            }
            n94 = case shown="False" w202 {
              tunnel: w210 -> [w384 w417]
              tunnel: w204 -> [w383 w414]
              tunnel: w209 -> [w382 _]
              tunnel: [w381 w413] -> w208
              tunnel: [w380 w417] -> w207
              tunnel: w203 -> [w379 _]
              frame False {
                n95 = case shown="True" w379 {
                  tunnel: w384 -> [w385 w404]
                  tunnel: w383 -> [w387 w403]
                  tunnel: w382 -> [_ w402]
                  tunnel: [w386 w391] -> w381
                  tunnel: [w385 w390] -> w380
                  frame False {
                    n96 = call "PADMINI_AUTO_BARCODE_STATUS.vi"("Enum"=enum16{"Read", "Write"}."Write", "error in (no error)"=w387, "I/P"=u16 2) -> ("error out"=w386:errorcluster)  [unwired: 7 in, 1 out]
                  }
                  frame True {
                    n97 = call "PADMINI_AUTO_BARCODE_STRING.vi"("Enum"=enum16{"Read", "Write"}."Read") -> ("Input 2"=w400:string)  [unwired: 9 in, 1 out]
                    n98 = Format Into String(format string="where BARCODE='%s'", w400) -> (resulting string=w397:string)  [unwired: 2 in, 1 out]
                    n99 = call <vilib>:"DB Tools Select Data.vi"("condition"=w397, "error in (no error)"=w403, "columns"=string[] ["BARCODE"], "table"=w402, "connection reference"=w404) -> ("error out"=w396:errorcluster, "data"=w395:variant[][], "connection reference out"=w390:T11)  [unwired: 1 in]
                    n100 = call "PADMINI_varient_to_data.vi"("error in (no error)"=w396, "data"=w395) -> ("error out"=w392:errorcluster, "Array"=w394:string[][])  [unwired: 8 in]
                    n101 = Empty Array?(array=w394) -> (empty?=w393:bool)
                    n102 = case shown="False" w393 {
                      tunnel: w392 -> [w408 w412]
                      tunnel: [w407 w409] -> w391
                      frame False {
                        n103 = call "PADMINI_AUTO_BARCODE_STATUS.vi"("Enum"=enum16{"Read", "Write"}."Write", "error in (no error)"=w408, "I/P"=u16 2) -> ("error out"=w407:errorcluster)  [unwired: 7 in, 1 out]
                      }
                      frame True {
                        n104 = call "PADMINI_AUTO_BARCODE_STATUS.vi"("Enum"=enum16{"Read", "Write"}."Write", "error in (no error)"=w412, "I/P"=u16 1) -> ("error out"=w409:errorcluster)  [unwired: 7 in, 1 out]
                      }
                    }
                  }
                }
              }
              frame True {
                n105 = call "PADMINI_AUTO_BARCODE_STATUS.vi"("Enum"=enum16{"Read", "Write"}."Write", "error in (no error)"=w414, "I/P"=u16 1) -> ("error out"=w413:errorcluster)  [unwired: 7 in, 1 out]
              }
            }
          }
          frame "SCAN2" {
            # "Barcode Status\n0-Ideal, 1-Ok, 2-Nok, 3-Prev Station Not Done,\n4-Prev Station Nok,\n5- Already Done"
            n106 = case shown="False" w423 {
              tunnel: w427 -> [w456 w564]
              tunnel: w426 -> [w448 w561]
              tunnel: w425 -> [_ _]
              tunnel: [w451 w560] -> w422
              tunnel: [w449 w564] -> w424
              frame False {
                # "2 FOR EMPTY BARCODE READ OR MISMATCH"
                # "0 = IF STATION 1 RESULT IS EMPTY\n1 = IF STATION 1 RESULT IS TRUE IS (LOGGED)\n       AND STATION 2 RESULT IS EMPTY (NOT LOGGED YET)\n2 = IF STATION 1 DATA IS LODDED BUT ITS FALSE(NOK)\n3 = IF STATION 2 RESULT IS STILL EMPTY ( YET NOT LOGGED)"
                n107 = global read "DATA LOG.vi" "OP30 ST 2 STRING"() -> (w433:string)
                n108 = call "PADMINI_AUTO_BARCODE_STRING2.vi"("Enum"=enum16{"Read", "Write"}."Read", "error in (no error)"=w448) -> ("error out"=w447:errorcluster)  [unwired: 8 in, 1 out]
                n109 = call <vilib>:"Trim Whitespace.vi"("string"=w433) -> ("trimmed string"=w432:string)  [unwired: 1 in]
                "trimmed string" <- w432
                n110 = disable-structure shown="Enabled" {
                  disable-tunnel: [w460 TRUE] -> w436
                  disable-tunnel: [w459 _] -> w435
                  disable-tunnel: [w457 _] -> w434
                  disable-tunnel: w432 -> [w458 _]
                  frame Enabled {
                    n111 = global read "Global 1.vi" "BARCODE RECIPE"() -> (w457:string)
                    n112 = Match Pattern(string=w458, regular expression=w457) -> (match substring=w459:string)  [unwired: 1 in, 3 out]
                    n113 = String Length(string=w457) -> (length=w462:i32)
                    n114 = String Length(string=w459) -> (length=w461:i32)
                    n115 = Equal?(x=w462, y=w461) -> (x = y?=w460:bool)
                  }
                  frame Disabled {
                  }
                }
                "match substring" <- w435
                "BARCODE RECIPE 2" <- w434
                n116 = String Length(string=w432) -> (length=→"length 2":i32)
                n117 = Format Into String(format string="WHERE BARCODE  ='%s'", w432) -> (resulting string=w443:string)  [unwired: 2 in, 1 out]
                n118 = call <vilib>:"DB Tools Select Data.vi"("condition"=w443, "error in (no error)"=w447, "columns"=string[] ["BARCODE", "ST1_RESULT", "ST2_RESULT"], "table"="REPORT", "connection reference"=w456) -> ("error out"=w454:errorcluster, "data"=w453:variant[][], "connection reference out"=w449:T11)  [unwired: 1 in]
                n119 = local read "OP 30"() -> (w442:T5)
                n120 = call "PADMINI_varient_to_data.vi"("error in (no error)"=w454, "data"=w453) -> ("error out"=w452:errorcluster, "Array"=w450:string[][])  [unwired: 8 in]
                n121 = Bundle By Name(cluster=w442, "BARCODE"=w432) -> (w441:T5)
                n122 = Equal?(x=w432, y="") -> (x = y?=w438:bool)
                n123 = local write "OP 30"(w441) -> ()
                n124 = call <userlib>:"Boolean Trigger__ogtk.vi"("Boolean Input"=w438) -> ("Rising Edge"=w440:bool)  [unwired: 1 in, 1 out]
                n125 = case shown="False" w438 {
                  selector: w438 -> [_ w559]
                  tunnel: w452 -> [w468 w557]
                  tunnel: [w467 w556] -> w451
                  tunnel: w450 -> [w466 _]
                  tunnel: w440 -> [w465 _]
                  tunnel: w436 -> [w464 _]
                  frame False {
                    n126 = case shown="True" w464 {
                      tunnel: w468 -> [w470 w485]
                      tunnel: [w469 w504] -> w467
                      tunnel: w466 -> [_ w503]
                      tunnel: w465 -> [_ w475]
                      frame False {
                        n127 = call "PADMINI_AUTO_BARCODE_STATUS2.vi"("Enum"=enum16{"Read", "Write"}."Write", "error in (no error)"=w470, "I/P"=u16 2) -> ("error out"=w469:errorcluster)  [unwired: 7 in, 1 out]
                      }
                      frame True {
                        # "ST2 RESULT"
                        # "ST1 RESULT"
                        n128 = Index Array(array=w503, index (row) #1=0 ("index (row)"), index (col) #1=1 ("disabled index (col)"), index (row) #2=0 ("index (row)"), index (col) #2=2 ("disabled index (col)")) -> (element #1=w481:string, element #2=w477:string)
                        n129 = Equal?(x=w481, y="OK") -> (x = y?=w482:bool)
                        n130 = call "READ OP30 RECHECK BIT.vi"("Enum"=enum16{"Read", "Write"}."Read", "error in (no error)"=w485) -> ("error out"=w484:errorcluster, "Input 2"=w490:dbl[])  [unwired: 8 in]
                        n131 = Not Equal?(x=w481, y="OK") -> (x != y?=w499:bool)
                        n132 = Empty String/Path?(string/path=w481) -> (empty?=w500:bool)
                        n133 = Empty String/Path?(string/path=w477) -> (empty?=w492:bool)
                        n134 = Equal?(x=w477, y="NOK") -> (x = y?=w474:bool)
                        n135 = And(x=w482, y=w492) -> (x .and. y?=w493:bool)
                        n136 = Equal?(x=w477, y="Aborted") -> (x = y?=w473:bool)
                        n137 = Not(x=w492) -> (.not. x?=w479:bool)
                        n138 = Index Array(array=w490, index=0) -> (element=w489:dbl)
                        n139 = Build Array(w500, w493, w499, w479, w475) -> (w498:bool[])
                        n140 = Equal?(x=w489, y=1.0) -> (x = y?=w483:bool)
                        n141 = Search 1D Array(1D array=w498, element=TRUE) -> (index of element=w496:i32)  [unwired: 1 in]
                        n142 = case shown="True" w483 {
                          tunnel: [w507 w534] -> w504
                          tunnel: w496 -> [w506 _]
                          tunnel: w484 -> [w505 w535]
                          tunnel: w474 -> [_ w533]
                          tunnel: w473 -> [_ w532]
                          frame False {
                            n143 = case shown="4" w506 {
                              tunnel: w505 -> [w509 w513 w519 w523 w527 w531]
                              tunnel: [w508 w512 w516 w520 w524 w528] -> w507
                              frame -1, Default {
                                n144 = call "PADMINI_AUTO_BARCODE_STATUS2.vi"("Enum"=enum16{"Read", "Write"}."Write", "error in (no error)"=w509, "I/P"=u16 0) -> ("error out"=w508:errorcluster)  [unwired: 7 in, 1 out]
                              }
                              frame 0 {
                                n145 = call "PADMINI_AUTO_BARCODE_STATUS2.vi"("Enum"=enum16{"Read", "Write"}."Write", "error in (no error)"=w513, "I/P"=u16 3) -> ("error out"=w512:errorcluster)  [unwired: 7 in, 1 out]
                              }
                              frame 1 {
                                n146 = call "PADMINI_AUTO_BARCODE_STATUS2.vi"("Enum"=enum16{"Read", "Write"}."Write", "error in (no error)"=w519, "I/P"=u16 1) -> ("error out"=w516:errorcluster)  [unwired: 7 in, 1 out]
                              }
                              frame 2 {
                                n147 = call "PADMINI_AUTO_BARCODE_STATUS2.vi"("Enum"=enum16{"Read", "Write"}."Write", "error in (no error)"=w523, "I/P"=u16 4) -> ("error out"=w520:errorcluster)  [unwired: 7 in, 1 out]
                              }
                              frame 3 {
                                n148 = call "PADMINI_AUTO_BARCODE_STATUS2.vi"("Enum"=enum16{"Read", "Write"}."Write", "error in (no error)"=w527, "I/P"=u16 5) -> ("error out"=w524:errorcluster)  [unwired: 7 in, 1 out]
                              }
                              frame 4 {
                                n149 = call "PADMINI_AUTO_BARCODE_STATUS2.vi"("Enum"=enum16{"Read", "Write"}."Write", "error in (no error)"=w531, "I/P"=u16 2) -> ("error out"=w528:errorcluster)  [unwired: 7 in, 1 out]
                              }
                            }
                          }
                          frame True {
                            n150 = case shown="False" w533 {
                              tunnel: w535 -> [w538 w552]
                              tunnel: [w537 w551] -> w534
                              tunnel: w532 -> [w536 _]
                              frame False {
                                n151 = case shown="True" w536 {
                                tunnel: w538 -> [w545 w548]
                                tunnel: [w539 w547] -> w537
                                frame False {
                                n152 = global write "Global 1.vi" "RECHECK RESULT OK"(TRUE ("RECHECK RESULT OK")) -> ()
                                n153 = call "RESET RECHECK OP40 BIT.vi"("Enum"=enum16{"Read", "Write"}."Write", "error in (no error)"=w545, "Array"=u16[] [0]) -> ("error out"=w540:errorcluster)  [unwired: 7 in, 1 out]
                                n154 = call "PADMINI_AUTO_BARCODE_STATUS2.vi"("Enum"=enum16{"Read", "Write"}."Write", "error in (no error)"=w540, "I/P"=u16 5) -> ("error out"=w539:errorcluster)  [unwired: 7 in, 1 out]
                                }
                                frame True {
                                n155 = call "PADMINI_AUTO_BARCODE_STATUS2.vi"("Enum"=enum16{"Read", "Write"}."Write", "error in (no error)"=w548, "I/P"=u16 1) -> ("error out"=w547:errorcluster)  [unwired: 7 in, 1 out]
                                }
                                }
                              }
                              frame True {
                                n156 = call "PADMINI_AUTO_BARCODE_STATUS2.vi"("Enum"=enum16{"Read", "Write"}."Write", "error in (no error)"=w552, "I/P"=u16 1) -> ("error out"=w551:errorcluster)  [unwired: 7 in, 1 out]
                              }
                            }
                          }
                        }
                        "Array" <- w503
                      }
                    }
                  }
                  frame True {
                    n157 = call "PADMINI_AUTO_BARCODE_STATUS2.vi"("Enum"=enum16{"Read", "Write"}."Write", "error in (no error)"=w557, "I/P"=u16 2) -> ("error out"=w556:errorcluster)  [unwired: 7 in, 1 out]
                    "OP30 BARCODE STRING EMPRTY" <- w559
                  }
                }
              }
              frame True {
                n158 = call "PADMINI_AUTO_BARCODE_STATUS2.vi"("Enum"=enum16{"Read", "Write"}."Write", "error in (no error)"=w561, "I/P"=u16 1) -> ("error out"=w560:errorcluster)  [unwired: 7 in, 1 out]
              }
            }
            n159 = flat-sequence {
              tunnel: [w431] -> w421
              tunnel: w422 -> [w431]
              frame #0 {
                n160 = local write "OP30 BARCODE STRING EMPRTY"(FALSE ("Boolean 5")) -> ()
                n161 = global write "DATA LOG.vi" "OP30 ST 2 STRING"("" ("OP30 ST 2 STRING")) -> ()
                n162 = global write "DATA LOG.vi" "scan op 30"(TRUE ("scan op 30")) -> ()
              }
            }
          }
          frame "SCAN3" {
            n163 = case shown="False" w569 {
              tunnel: w573 -> [w599 w689]
              tunnel: w572 -> [w598 w687]
              tunnel: w571 -> [w597 _]
              tunnel: [w588 w686] -> w568
              tunnel: [w591 w689] -> w570
              frame False {
                # "Barcode Status\n0-Ideal, 1-Ok, 2-Nok, 3-Prev Station Not Done,\n4-Prev Station Nok,\n5- Already Done"
                # "0 = IF STATION 1 RESULT IS EMPTY\n1 = IF STATION 1 RESULT IS TRUE IS (LOGGED)\n       AND STATION 2 RESULT IS EMPTY (NOT LOGGED YET)\n2 = IF STATION 1 DATA IS LODDED BUT ITS FALSE(NOK)\n3 = IF STATION 2 RESULT IS STILL EMPTY ( YET NOT LOGGED)"
                n164 = global read "DATA LOG.vi" "ST 3 STRING 2"() -> (w586:string)
                n165 = local read "OP 40"() -> (w583:T7)
                n166 = call <vilib>:"Trim Whitespace.vi"("string"=w586) -> ("trimmed string"=w581:string)  [unwired: 1 in]
                n167 = disable-structure shown="Enabled" {
                  disable-tunnel: w581 -> [w601 _]
                  disable-tunnel: [w602 TRUE] -> w580
                  frame Enabled {
                    (unwired) "False"
                    (unwired) "True"
                    n168 = global read "Global 1.vi" "BARCODE RECIPE"() -> (w600:string)
                    n169 = Match Pattern(string=w601, regular expression=w600) -> (match substring=w605:string)  [unwired: 1 in, 3 out]
                    n170 = String Length(string=w600) -> (length=w604:i32)
                    n171 = String Length(string=w605) -> (length=w603:i32)
                    n172 = Equal?(x=w604, y=w603) -> (x = y?=w602:bool)
                  }
                  frame Disabled {
                  }
                }
                n173 = Bundle By Name(cluster=w583, "BARCODE"=w581) -> (w582:T7)
                n174 = Format Into String(format string="where BARCODE='%s'", w581) -> (resulting string=w594:string)  [unwired: 2 in, 1 out]
                n175 = call <vilib>:"DB Tools Select Data.vi"("condition"=w594, "error in (no error)"=w598, "columns"=string[] ["BARCODE", "ST2_RESULT", "ST3_RESULT"], "table"=w597, "connection reference"=w599) -> ("error out"=w593:errorcluster, "data"=w592:variant[][], "connection reference out"=w591:T11)  [unwired: 1 in]
                n176 = Equal?(x=w581, y="") -> (x = y?=w584:bool)
                n177 = local write "OP 40"(w582) -> ()
                n178 = case shown="False" w584 {
                  selector: w584 -> [_ w684]
                  tunnel: w593 -> [w611 w682]
                  tunnel: w592 -> [w610 _]
                  tunnel: [w609 w682] -> w589
                  tunnel: [w608 2] -> w587
                  tunnel: w580 -> [w607 _]
                  frame False {
                    n179 = case shown="True" w607 {
                      tunnel: w611 -> [w612 w648]
                      tunnel: w610 -> [_ w647]
                      tunnel: [w612 w638] -> w609
                      tunnel: [u16 2 ("I/P") w637] -> w608
                      frame False {
                      }
                      frame True {
                        (unwired) "OK"
                        (unwired) "OK"
                        n180 = call "PADMINI_varient_to_data.vi"("error in (no error)"=w648, "data"=w647) -> ("error out"=w619:errorcluster, "Array"=w639:string[][])  [unwired: 8 in]
                        n181 = Index Array(array=w639, index (row) #1=0 ("index (row)"), index (col) #1=1 ("disabled index (col)"), index (row) #2=0 ("index (row)"), index (col) #2=2 ("disabled index (col)")) -> (element #1=w622:string, element #2=w616:string)
                        n182 = call <vilib>:"Clear Errors.vi"("error in (no error)"=w619) -> ("error out"=w618:errorcluster)  [unwired: 5 in, 1 out]
                        n183 = Not Equal?(x=w622, y="OK") -> (x != y?=w645:bool)
                        n184 = Equal?(x=w622, y="OK") -> (x = y?=w624:bool)
                        n185 = Empty String/Path?(string/path=w622) -> (empty?=w646:bool)
                        n186 = Empty String/Path?(string/path=w616) -> (empty?=w640:bool)
                        n187 = call "RECHECK READ BIT.vi"("Enum"=enum16{"Read", "Write"}."Read", "error in (no error)"=w618) -> ("error out"=w625:errorcluster, "Input 2"=w629:dbl[])  [unwired: 8 in]
                        n188 = Equal?(x=w616, y="Aborted") -> (x = y?=w614:bool)
                        n189 = Equal?(x=w616, y="NOK") -> (x = y?=w615:bool)
                        n190 = And(x=w624, y=w640) -> (x .and. y?=w641:bool)
                        n191 = Not(x=w640) -> (.not. x?=w636:bool)
                        n192 = Index Array(array=w629, index=0) -> (element=w630:dbl)
                        n193 = Build Array(w646, w641, w645, w636) -> (w644:bool[])
                        n194 = Equal?(x=w630, y=1.0) -> (x = y?=w620:bool)
                        n195 = Search 1D Array(1D array=w644, element=TRUE) -> (index of element=w642:i32)  [unwired: 1 in]
                        n196 = case shown="True" w620 {
                          tunnel: w642 -> [w652 _]
                          tunnel: [w651 w664] -> w638
                          tunnel: [w650 w667] -> w637
                          tunnel: w625 -> [w649 w665]
                          tunnel: w615 -> [_ w666]
                          tunnel: w614 -> [_ w663]
                          frame False {
                            n197 = case shown="3" w652 {
                              tunnel: [w654 w655 w657 w659 w662] -> w651
                              tunnel: w649 -> [w654 w655 w657 w659 w662]
                              tunnel: [u16 0 ("I/P") u16 3 ("I/P") u16 1 ("I/P") u16 4 ("I/P") u16 5 ("I/P")] -> w650
                              frame -1, Default {
                              }
                              frame 0 {
                              }
                              frame 1 {
                              }
                              frame 2 {
                              }
                              frame 3 {
                              }
                            }
                          }
                          frame True {
                            n198 = case shown="False" w666 {
                              tunnel: [w671 u16 1 ("I/P")] -> w667
                              tunnel: w665 -> [w670 w680]
                              tunnel: [w669 w680] -> w664
                              tunnel: w663 -> [w668 _]
                              frame False {
                                n199 = case shown="False" w668 {
                                tunnel: [u16 5 ("I/P") u16 1 ("I/P")] -> w671
                                tunnel: w670 -> [w673 w679]
                                tunnel: [w672 w679] -> w669
                                frame False {
                                n200 = global write "Global 1.vi" "RECHECK RESULT OK"(TRUE ("RECHECK RESULT OK")) -> ()
                                n201 = call "SEND RECHECK ABORT BUTTON.vi"("Enum"=enum16{"Read", "Write"}."Write", "error in (no error)"=w673, "Array"=u16[] [0]) -> ("error out"=w672:errorcluster)  [unwired: 7 in, 1 out]
                                }
                                frame True {
                                }
                                }
                              }
                              frame True {
                              }
                            }
                          }
                        }
                      }
                    }
                  }
                  frame True {
                    "OP40 BARCODE STRING EMPRTY" <- w684
                  }
                }
                n202 = call "PADMINI_AUTO_BARCODE_STATUS3.vi"("Enum"=enum16{"Read", "Write"}."Write", "error in (no error)"=w589, "I/P"=w587) -> ("error out"=w588:errorcluster)  [unwired: 7 in, 1 out]
              }
              frame True {
                n203 = call "PADMINI_AUTO_BARCODE_STATUS3.vi"("Enum"=enum16{"Read", "Write"}."Write", "error in (no error)"=w687, "I/P"=u16 1) -> ("error out"=w686:errorcluster)  [unwired: 7 in, 1 out]
              }
            }
            n204 = flat-sequence {
              tunnel: [w579] -> w567
              tunnel: w568 -> [w579]
              frame #0 {
                n205 = local write "OP40 BARCODE STRING EMPRTY"(FALSE) -> ()
                n206 = global write "DATA LOG.vi" "scan op 40"(TRUE ("scan op 40")) -> ()
                n207 = global write "DATA LOG.vi" "ST 3 STRING 2"("" ("ST 3 STRING 2")) -> ()
                n208 = global write "DATA LOG.vi" "op 40"(0 ("op 30")) -> ()
              }
            }
          }
          frame "SCAN4" {
            # "AC300711701GGN/PRCV241221045"
            # "Barcode Status\n0-Ideal, \n1-Ok, 2-Nok, 3-Prev Station Not Done,\n4-Prev Station Nok,\n5- Already Done"
            n209 = case shown="False" w696 {
              tunnel: w700 -> [w742 w878]
              tunnel: w699 -> [w726 w877]
              tunnel: w698 -> [w741 _]
              tunnel: [w732 w876] -> w694
              tunnel: [w734 w878] -> w697
              tunnel: w693 -> [w722 w873]
              tunnel: [w721 w873] -> w692
              tunnel: [w708 w872] -> w691
              tunnel: w690 -> [w713 w872]
              frame False {
                # "0 = IF STATION 1 RESULT IS EMPTY\n1 = IF STATION 1 RESULT IS TRUE IS (LOGGED)\n       AND STATION 2 RESULT IS EMPTY (NOT LOGGED YET)\n2 = IF STATION 1 DATA IS LODDED BUT ITS FALSE(NOK)\n3 = IF STATION 2 RESULT IS STILL EMPTY ( YET NOT LOGGED)"
                # "STATION 4 BARCODE STRING"
                n210 = global read "DATA LOG.vi" "ST 4 STRING 3"() -> (w716:string)
                "scanner value" <- w716
                n211 = Empty String/Path?(string/path=w716) -> (empty?=w718:bool)
                n212 = call "PADMINI_AUTO_BARCODE_STRING4.vi"("Enum"=enum16{"Read", "Write"}."Read", "error in (no error)"=w726) -> ("error out"=w725:errorcluster)  [unwired: 8 in, 1 out]
                n213 = Not(x=w718) -> (.not. x?=w719:bool)
                n214 = call <vilib>:"Trim Whitespace.vi"("string"=w716) -> ("trimmed string"=w708:string)  [unwired: 1 in]
                n215 = disable-structure shown="Enabled" {
                  disable-tunnel: "" -> [w870 _]
                  disable-tunnel: [w869 _] -> w727
                  disable-tunnel: w708 -> [w864 _]
                  disable-tunnel: [w865 TRUE] -> w720
                  frame Enabled {
                    n216 = global read "Global 1.vi" "BARCODE RECIPE"() -> (w863:string)
                    n217 = Match Pattern(string=w864, regular expression=w863) -> (match substring=w868:string)  [unwired: 1 in, 3 out]
                    n218 = String Length(string=w863) -> (length=w867:i32)
                    n219 = String Length(string=w868) -> (length=w866:i32)
                    n220 = Equal?(x=w864, y=w870) -> (x = y?=w869:bool)
                    n221 = Equal?(x=w867, y=w866) -> (x = y?=w865:bool)
                  }
                  frame Disabled {
                  }
                }
                n222 = Equal?(x=w713, y=w708) -> (x = y?=w712:bool)
                n223 = call-poly <userlib>:"Data Changed__ogtk.vi"("String"=w716) -> ("Changed"=w717:bool)
                n224 = Equal?(x=w708, y="ERROR") -> (x = y?=w710:bool)
                n225 = And(x=w717, y=w719) -> (x .and. y?=w715:bool)
                n226 = global write "Global 1.vi" "OP 60 BARCODE"(w708) -> ()
                n227 = local read "OP 60"() -> (w729:T8)
                n228 = Bundle By Name(cluster=w729, "BARCODE"=w708) -> (w723:T8)
                n229 = String To Byte Array(string=w708) -> (unsigned byte array=w724:u8[])
                n230 = Or(x=w712, y=w710) -> (x .or. y?=w709:bool)
                n231 = Format Into String(format string="where BARCODE='%s'", w708) -> (resulting string=w737:string)  [unwired: 2 in, 1 out]
                n232 = Not(x=w715) -> (.not. x?=w714:bool)
                n233 = global write "DATA LOG.vi" "string to bye array"(w724) -> ()
                n234 = global write "DATA LOG.vi" "test barcode"(w708) -> ()
                n235 = call <vilib>:"DB Tools Select Data.vi"("condition"=w737, "error in (no error)"=w725, "columns"=string[] ["BARCODE", "ST3_RESULT", "ST4_RESULT"], "table"=w741, "connection reference"=w742) -> ("error out"=w736:errorcluster, "data"=w735:variant[][], "connection reference out"=w734:T11)  [unwired: 1 in]
                n236 = local write "OP 61"(w723) -> ()
                n237 = local write "OP 60"(w723) -> ()
                n238 = case shown="False" w709 {
                  tunnel: w736 -> [w752 w860]
                  tunnel: w735 -> [w751 _]
                  tunnel: [w750 w859] -> w733
                  tunnel: [w749 u16 2 ("I/P")] -> w730
                  tunnel: w727 -> [w748 _]
                  tunnel: w722 -> [w747 w861]
                  tunnel: [w746 w861] -> w721
                  tunnel: w720 -> [w745 _]
                  tunnel: w714 -> [w744 _]
                  tunnel: w708 -> [w743 _]
                  frame False {
                    n239 = case shown="True" w748 {
                      selector: w748 -> [_ w852]
                      tunnel: w752 -> [w761 w851]
                      tunnel: w751 -> [w760 _]
                      tunnel: [w759 w850] -> w750
                      tunnel: [w758 u16 2 ("I/P")] -> w749
                      tunnel: w743 -> [w757 _]
                      tunnel: w747 -> [w756 w848]
                      tunnel: [w755 w848] -> w746
                      tunnel: w745 -> [w754 _]
                      tunnel: w744 -> [w753 _]
                      frame False {
                        n240 = case shown="True" w754 {
                          tunnel: w761 -> [w762 w803]
                          tunnel: w760 -> [_ w802]
                          tunnel: [w762 w792] -> w759
                          tunnel: [u16 2 ("I/P") w791] -> w758
                          tunnel: w757 -> [_ w784]
                          tunnel: w756 -> [w764 w783]
                          tunnel: [w764 w782] -> w755
                          tunnel: w753 -> [_ _]
                          frame False {
                          }
                          frame True {
                            n241 = call "PADMINI_varient_to_data.vi"("error in (no error)"=w803, "data"=w802) -> ("error out"=w772:errorcluster, "Array"=w793:string[][])  [unwired: 8 in]
                            n242 = Index Array(array=w793, index (row) #1=0 ("index (row)"), index (col) #1=1 ("disabled index (col)"), index (row) #2=0 ("index (row)"), index (col) #2=2 ("disabled index (col)")) -> (element #1=w774:string, element #2=w767:string)
                            n243 = call <vilib>:"Clear Errors.vi"("error in (no error)"=w772) -> ("error out"=w771:errorcluster)  [unwired: 5 in, 1 out]
                            n244 = Not Equal?(x=w774, y="OK") -> (x != y?=w800:bool)
                            n245 = Equal?(x=w774, y="OK") -> (x = y?=w796:bool)
                            n246 = Empty String/Path?(string/path=w774) -> (empty?=w801:bool)
                            n247 = Empty String/Path?(string/path=w767) -> (empty?=w794:bool)
                            n248 = call "READ OP60 RECHECK BIT.vi"("Enum"=enum16{"Read", "Write"}."Read", "error in (no error)"=w771) -> ("error out"=w766:errorcluster, "Input 2"=w780:dbl[])  [unwired: 8 in]
                            n249 = And(x=w796, y=w794) -> (x .and. y?=w795:bool)
                            n250 = Not(x=w794) -> (.not. x?=w790:bool)
                            n251 = Equal?(x=w767, y="NOK") -> (x = y?=w769:bool)
                            n252 = Equal?(x=w767, y="Aborted") -> (x = y?=w768:bool)
                            n253 = Index Array(array=w780, index=0) -> (element=w778:dbl)
                            n254 = Build Array(w801, w795, w800, w790) -> (w799:bool[])
                            n255 = Equal?(x=w778, y=1.0) -> (x = y?=w776:bool)
                            n256 = Search 1D Array(1D array=w799, element=TRUE) -> (index of element=w797:i32)  [unwired: 1 in]
                            n257 = call <vilib>:"Clear Errors.vi"("error in (no error)"=w766) -> ("error out"=w765:errorcluster)  [unwired: 5 in, 1 out]
                            n258 = case shown="True" w776 {
                              tunnel: w797 -> [w810 _]
                              tunnel: w765 -> [w809 w831]
                              tunnel: [w808 w830] -> w792
                              tunnel: [w807 w833] -> w791
                              tunnel: w784 -> [w806 _]
                              tunnel: w783 -> [w805 w832]
                              tunnel: [w804 w832] -> w782
                              tunnel: w769 -> [_ w829]
                              tunnel: w768 -> [_ w828]
                              frame False {
                                n259 = case shown="2" w810 {
                                tunnel: [w813 w815 w820 w823 w827] -> w808
                                tunnel: w809 -> [w813 w815 w820 w823 w827]
                                tunnel: [u16 2 ("I/P") u16 3 ("I/P") u16 1 ("I/P") u16 4 ("I/P") u16 5 ("I/P")] -> w807
                                tunnel: w806 -> [_ _ w819 _ _]
                                tunnel: w805 -> [w811 w814 w818 w822 w825]
                                tunnel: [w811 w814 w817 w822 w825] -> w804
                                frame -1 {
                                }
                                frame 0 {
                                }
                                frame 1, Default {
                                n260 = Build Array (concatenate)(w818, w819) -> (w817:string[])
                                }
                                frame 2 {
                                }
                                frame 3 {
                                }
                                }
                              }
                              frame True {
                                n261 = case shown="False" w829 {
                                tunnel: [w837 u16 1 ("I/P")] -> w833
                                tunnel: [w835 w847] -> w830
                                tunnel: w831 -> [w836 w847]
                                tunnel: w828 -> [w834 _]
                                frame False {
                                n262 = case shown="True" w834 {
                                tunnel: [u16 5 ("I/P") u16 1 ("I/P")] -> w837
                                tunnel: w836 -> [w839 w844]
                                tunnel: [w838 w844] -> w835
                                frame False {
                                n263 = global write "Global 1.vi" "RECHECK RESULT OK"(TRUE ("RECHECK RESULT OK")) -> ()
                                n264 = call "RESET RECHECK OP60 BIT.vi"("Enum"=enum16{"Read", "Write"}."Write", "error in (no error)"=w839, "Array"=u16[] [0]) -> ("error out"=w838:errorcluster)  [unwired: 7 in, 1 out]
                                }
                                frame True {
                                }
                                }
                                }
                                frame True {
                                }
                                }
                              }
                            }
                          }
                        }
                      }
                      frame True {
                        n265 = disable-structure shown="Enabled" {
                          disable-tunnel: w851 -> [w856 w858]
                          disable-tunnel: [w855 w857] -> w850
                          frame Disabled {
                            n266 = call "PADMINI_AUTO_BARCODE_STATUS4.vi"("Enum"=enum16{"Read", "Write"}."Write", "error in (no error)"=w856, "I/P"=u16 2) -> ("error out"=w855:errorcluster)  [unwired: 7 in, 1 out]
                          }
                          frame Enabled {
                            n267 = call <vilib>:"Clear Errors.vi"("error in (no error)"=w858) -> ("error out"=w857:errorcluster)  [unwired: 5 in, 1 out]
                          }
                        }
                        "Boolean 5" <- w852
                      }
                    }
                  }
                  frame True {
                    n268 = call <vilib>:"Clear Errors.vi"("error in (no error)"=w860) -> ("error out"=w859:errorcluster)  [unwired: 5 in, 1 out]
                  }
                }
                n269 = call "PADMINI_AUTO_BARCODE_STATUS4.vi"("Enum"=enum16{"Read", "Write"}."Write", "error in (no error)"=w733, "I/P"=w730) -> ("error out"=w732:errorcluster)  [unwired: 7 in, 1 out]
                "PRIVIOUS DATA" <- w713
              }
              frame True {
                n270 = call "PADMINI_AUTO_BARCODE_STATUS4.vi"("Enum"=enum16{"Read", "Write"}."Write", "error in (no error)"=w877, "I/P"=u16 1) -> ("error out"=w876:errorcluster)  [unwired: 7 in, 1 out]
              }
            }
            n271 = flat-sequence {
              tunnel: [w705] -> w695
              tunnel: w694 -> [w706]
              frame #0 {
                n272 = call "PADMINI_AUTO_BARCODE_STRING4.vi"("Enum"=enum16{"Read", "Write"}."Write", "error in (no error)"=w706, "Input"="" ("ST 4 STRING 3")) -> ("error out"=w705:errorcluster)  [unwired: 7 in, 1 out]
                n273 = local write "Boolean 5"(TRUE ("Boolean 5")) -> ()
                n274 = global write "DATA LOG.vi" "scan op 60"(TRUE ("scan op 60")) -> ()
              }
            }
          }
          frame "DATALOG1" {
            w882 = T12 2 items=["no dialog", "OK message", "continue or stop message", "OK message + warnings", "continue/stop + warnings"] ("type of dialog (OK msg:1)")
            # "cycle result status\nwhether it was ok or nok\nor abortted in between"
            # "Printed QR Code data string"
            # "datalog of st 1"
            n275 = local read "STATION-1 2"() -> (w925:T4)
            n276 = call "PADMINI_AUTO_CYCLE STATE.vi"("Enum"=enum16{"Read", "Write"}."Read", "error in (no error)"=w893) -> ("error out"=w892:errorcluster, "Input 2"=w890:u16[])  [unwired: 8 in]
            n277 = call "PADMINI_AUTO_BARCODE_STRING.vi"("Enum"=enum16{"Read", "Write"}."Read") -> ("Input 2"=w885:string)  [unwired: 9 in, 1 out]
            n278 = Unbundle By Name(w925) -> ("OK PART"=w917:dbl, "NOK PART"=w916:dbl, "TOTAL"=w915:dbl, "CYCLE TIME"=w924:dbl, "PARAMETER 1"=w923:dbl, "PARAMETER 2"=w922:dbl, "PARAMETER 3"=w921:dbl, "PARAMETER 4"=w920:dbl, "PARAMETER 5"=w919:dbl, "PARAMETER 6"=w918:dbl, "SCANNER"=w914:bool, "CYCLE STATUS"=w913:bool, "PARAMETER 1"=w912:bool, "PARAMETER 2"=w911:bool, "PARAMETER 3"=w910:bool, "PARAMETER 5"=w899:bool, "PARAMETER 7"=w898:bool, "CYCLE RESULT"=w897:bool)  [unwired: 6 out]
            n279 = Index Array(array=w890, index=2) -> (element=w895:u16)
            n280 = disable-structure shown="Enabled" {
              disable-tunnel: [w930 w932] -> w886
              disable-tunnel: w885 -> [w929 w932]
              frame Disabled {
                n281 = String Length(string=w929) -> (length=w928:i32)
                n282 = Decrement(x=w928) -> (x-1=w927:i32)
                n283 = String Subset(string=w929, offset (0)=0, length (rest)=w927) -> (substring=w930:string)
              }
              frame Enabled {
              }
            }
            n284 = case shown="3" w895 {
              tunnel: ["" "OK" "NOK" "Aborted"] -> w894
              frame 0 {
              }
              frame 1, Default {
              }
              frame 2 {
              }
              frame 3 {
              }
            }
            n285 = Build Array(w917, w916, w915, w924, w923, w922, w921, w920, w919, w918) -> (w906:dbl[])
            n286 = Build Array(w914, w913, w912, w911, w910, w899, w898) -> (w905:bool[])
            n287 = call <vilib>:"Trim Whitespace.vi"("string"=w886) -> ("trimmed string"=w887:string)  [unwired: 1 in]
            n288 = String Length(string=w887) -> (length=→"length":i32)
            n289 = case shown="False" w908 {
              tunnel: w909 -> [w950 w989]
              tunnel: w892 -> [w952 w988]
              tunnel: [w960 w987] -> w904
              tunnel: [w959 w986] -> w883
              tunnel: w907 -> [w947 _]
              tunnel: w887 -> [w944 _]
              tunnel: w906 -> [w956 w982]
              tunnel: w905 -> [w955 w981]
              tunnel: w897 -> [_ w977]
              tunnel: w894 -> [w954 w976]
              frame False {
                w946 = string[] ["BARCODE", "SHIFT", "DATE", "ST1_REAL_DATA", "ST1_BOOL_DATA", "ST1_RESULT"]
                # "ST1 RESULT"
                n290 = local read "SHIFT"() -> (w958:string)
                n291 = Format Into String(format string="Where BARCODE='%s' ", w944) -> (resulting string=w939:string)  [unwired: 2 in, 1 out]
                n292 = call <vilib>:"DB Tools Select Data.vi"("condition"=w939, "error in (no error)"=w952, "columns"=w946, "table"=w947, "connection reference"=w950) -> ("error out"=w948:errorcluster, "data"=w951:variant[][], "connection reference out"=w949:T11)  [unwired: 1 in]
                n293 = call "PADMINI_SHIFT_DATE.vi"("SHIFT"=w958) -> ("date/time string"=w957:string)  [unwired: 10 in]
                n294 = Variant To Data(error in=w948, type=string[][] [], Variant=w951) -> (data=w942:string[][], error out=w940:errorcluster)
                n295 = Bundle("trimmed string"=w944, "SHIFT"=w958, "date/time string"=w957, w956, w955, w954) -> (w953:T13)  [unwired: 1 in]
                n296 = Empty Array?(array=w942) -> (empty?=w941:bool)
                n297 = case shown="False" w941 {
                  tunnel: w949 -> [w965 w975]
                  tunnel: w940 -> [w964 w974]
                  tunnel: [w968 w973] -> w960
                  tunnel: [w967 w972] -> w959
                  tunnel: w946 -> [w962 w971]
                  tunnel: w947 -> [w963 w970]
                  tunnel: w953 -> [w966 w969]
                  tunnel: w939 -> [w961 _]
                  frame False {
                    n298 = call <vilib>:"DB Tools Update Data.vi"("condition"=w961, "data"=w966, "error in (no error)"=w964, "columns"=w962, "table"=w963, "connection reference"=w965) -> ("error out"=w967:errorcluster, "connection reference out"=w968:T11)  [unwired: 4 in]
                  }
                  frame True {
                    n299 = call <vilib>:"DB Tools Insert Data.vi"("data"=w969, "error in (no error)"=w974, "columns"=w971, "table"=w970, "connection reference"=w975) -> ("error out"=w972:errorcluster, "connection reference out"=w973:T11)  [unwired: 5 in]
                  }
                }
              }
              frame True {
                n300 = local read "SHIFT"() -> (w984:string)
                n301 = call "PADMINI_SHIFT_DATE.vi"("SHIFT"=w984) -> ("date/time string"=w983:string)  [unwired: 10 in]
                n302 = Bundle("SHIFT"=w984, "date/time string"=w983, w982, w981, "CYCLE RESULT"=w977, w976) -> (w980:T14)  [unwired: 1 in]
                n303 = To Variant(anything=w980) -> (Variant=w979:variant)
                n304 = call <vilib>:"DB Tools Insert Data.vi"("data"=w979, "error in (no error)"=w988, "columns"=string[] ["SHIFT", "DATE", "ST1_REAL_DATA", "ST1_BOOL_DATA", "ST1_RESULT", "RESULT"], "table"="ST1_REPORT", "connection reference"=w989) -> ("error out"=w986:errorcluster, "connection reference out"=w987:T11)  [unwired: 5 in]
              }
            }
            n305 = call <vilib>:"Simple Error Handler.vi"("type of dialog (OK msg:1)"=w882, "error in (no error)"=w883) -> ("error out"=w881:errorcluster)  [unwired: 3 in, 4 out]
            n306 = call <vilib>:"Clear Errors.vi"("error in (no error)"=w881) -> ("error out"=w880:errorcluster)  [unwired: 5 in, 1 out]
            n307 = flat-sequence {
              tunnel: [w937] -> w900
              tunnel: w901 -> [w937]
              frame #0 {
                n308 = global write "DATA LOG.vi" "DATA LOG RESET"(TRUE ("DATA LOG RESET")) -> ()
              }
            }
            n309 = call "PADMINI_AUTO_DATALOG_DONE.vi"("Enum"=enum16{"Read", "Write"}."Write", "error in (no error)"=w880, "I/P"=u16 2) -> ("error out"=w901:errorcluster)  [unwired: 7 in, 1 out]
          }
          frame "DATALOG2" {
            w991 = T12 2 items=["no dialog", "OK message", "continue or stop message", "OK message + warnings", "continue/stop + warnings"] ("type of dialog (OK msg:1)")
            # "ST2_REAL_DATA\nST2_BOOL_DATA\nDATE\nSHIFT"
            # "datalog of st 2"
            n310 = local read "STATION-2 2"() -> (w1025:T3)
            n311 = call "PADMINI_AUTO_CYCLE STATE2.vi"("Enum"=enum16{"Read", "Write"}."Read", "error in (no error)"=w997) -> ("error out"=w996:errorcluster, "Input 2"=w1000:u16[])  [unwired: 8 in]
            n312 = Unbundle By Name(w1025) -> ("BARCODE"=w1011:string, "OK PART"=w1021:dbl, "NOK PART"=w1020:dbl, "TOTAL"=w1019:dbl, "CYCLE TIME"=w1024:dbl, "PARAMETER 1"=w1023:dbl, "PARAMETER 2"=w1022:dbl, "SCANNER"=w1018:bool, "CYCLE STATUS"=w1017:bool, "PARAMETER 1"=w1016:bool, "PARAMETER 2"=w1015:bool, "CYCLE RESULT"=w1003:bool)  [unwired: 9 out]
            n313 = Index Array(array=w1000, index=2) -> (element=w999:u16)
            n314 = case shown="3" w999 {
              tunnel: ["" "OK" "NOK" "Aborted"] -> w998
              frame 0 {
              }
              frame 1, Default {
              }
              frame 2 {
              }
              frame 3 {
              }
            }
            n315 = Build Array(w1021, w1020, w1019, w1024, w1023, w1022) -> (w1010:dbl[])
            n316 = Build Array(w1018, w1017, w1016, w1015) -> (w1009:bool[])
            n317 = case shown="False" w1013 {
              tunnel: w1014 -> [w1047 w1061]
              tunnel: w996 -> [w1046 w1060]
              tunnel: [w1045 w1059] -> w1008
              tunnel: [w1044 w1058] -> w993
              tunnel: w1012 -> [w1043 _]
              tunnel: w1011 -> [w1037 _]
              tunnel: w1010 -> [w1040 w1054]
              tunnel: w1009 -> [w1035 w1053]
              tunnel: w1003 -> [_ w1049]
              tunnel: w998 -> [w1033 w1048]
              frame False {
                n318 = local read "SHIFT"() -> (w1042:string)
                n319 = call "PADMINI_SHIFT_DATE.vi"("SHIFT"=w1042) -> ("date/time string"=w1041:string)  [unwired: 10 in]
                n320 = Bundle("SHIFT"=w1042, "date/time string"=w1041, w1040, w1035, w1033) -> (w1034:T15)  [unwired: 1 in]
                n321 = To Variant(anything=w1034) -> ()  [unwired: 1 out]
                n322 = Format Into String(format string="where BARCODE='%s'", w1037) -> (resulting string=w1036:string)  [unwired: 2 in, 1 out]
                n323 = call <vilib>:"DB Tools Update Data.vi"("condition"=w1036, "data"=w1034, "error in (no error)"=w1046, "columns"=string[] ["SHIFT", "DATE", "ST2_REAL_DATA", "ST2_BOOL_DATA", "ST2_RESULT"], "table"=w1043, "connection reference"=w1047) -> ("error out"=w1044:errorcluster, "connection reference out"=w1045:T11)  [unwired: 4 in]
              }
              frame True {
                n324 = local read "SHIFT"() -> (w1056:string)
                n325 = call "PADMINI_SHIFT_DATE.vi"("SHIFT"=w1056) -> ("date/time string"=w1055:string)  [unwired: 10 in]
                n326 = Bundle("SHIFT"=w1056, "date/time string"=w1055, w1054, w1053, "CYCLE RESULT"=w1049, w1048) -> (w1052:T14)  [unwired: 1 in]
                n327 = To Variant(anything=w1052) -> (Variant=w1051:variant)
                n328 = call <vilib>:"DB Tools Insert Data.vi"("data"=w1051, "error in (no error)"=w1060, "columns"=string[] ["SHIFT", "DATE", "ST2_REAL_DATA", "ST2_BOOL_DATA", "ST2_RESULT", "RESULT"], "table"="ST2_REPORT", "connection reference"=w1061) -> ("error out"=w1058:errorcluster, "connection reference out"=w1059:T11)  [unwired: 5 in]
              }
            }
            n329 = call <vilib>:"Simple Error Handler.vi"("type of dialog (OK msg:1)"=w991, "error in (no error)"=w993) -> ("error out"=w994:errorcluster)  [unwired: 3 in, 4 out]
            n330 = call <vilib>:"Clear Errors.vi"("error in (no error)"=w994) -> ("error out"=w992:errorcluster)  [unwired: 5 in, 1 out]
            n331 = flat-sequence {
              tunnel: [w1031] -> w1004
              tunnel: w1005 -> [w1031]
              frame #0 {
                n332 = global write "DATA LOG.vi" "DATA LOG RESET 2"(TRUE ("DATA LOG RESET")) -> ()
              }
            }
            n333 = call "PADMINI_AUTO_DATALOG_DONE2.vi"("Enum"=enum16{"Read", "Write"}."Write", "error in (no error)"=w992, "I/P"=u16 2) -> ("error out"=w1005:errorcluster)  [unwired: 7 in, 1 out]
          }
          frame "DATALOG3" {
            w1064 = T12 2 items=["no dialog", "OK message", "continue or stop message", "OK message + warnings", "continue/stop + warnings"] ("type of dialog (OK msg:1)")
            # "ST3_REAL_DATA\nST3_BOOL_DATA\nDATE\nSHIFT"
            # "datalog of st 3"
            n334 = local read "STATION-3 2"() -> (w1107:T3)
            n335 = call "PADMINI_AUTO_CYCLE STATE3.vi"("Enum"=enum16{"Read", "Write"}."Read", "error in (no error)"=w1071) -> ("error out"=w1070:errorcluster, "Input 2"=w1072:u16[])  [unwired: 8 in]
            n336 = Unbundle By Name(w1107) -> ("BARCODE"=w1083:string, "OK PART"=w1098:dbl, "NOK PART"=w1097:dbl, "TOTAL"=w1096:dbl, "CYCLE TIME"=w1106:dbl, "PARAMETER 1"=w1105:dbl, "PARAMETER 2"=w1104:dbl, "PARAMETER 3"=w1103:dbl, "PARAMETER 4"=w1102:dbl, "PARAMETER 5"=w1101:dbl, "PARAMETER 6"=w1100:dbl, "PARAMETER 7"=w1099:dbl, "SCANNER"=w1095:bool, "CYCLE STATUS"=w1094:bool, "PARAMETER 1"=w1093:bool, "PARAMETER 2"=w1092:bool, "PARAMETER 3"=w1091:bool, "PARAMETER 4"=w1090:bool, "PARAMETER 5"=w1089:bool, "PARAMETER 6"=w1088:bool, "PARAMETER 7"=w1087:bool, "CYCLE RESULT"=w1076:bool)  [unwired: 4 out]
            n337 = Index Array(array=w1072, index=2) -> (element=w1074:u16)
            n338 = case shown="2" w1074 {
              tunnel: ["" "OK" "NOK" "Aborted"] -> w1069
              frame 0 {
              }
              frame 1, Default {
              }
              frame 2 {
              }
              frame 3 {
              }
            }
            n339 = Build Array(w1098, w1097, w1096, w1106, w1105, w1104, w1103, w1102, w1101, w1100, w1099) -> (w1082:dbl[])
            n340 = Build Array(w1095, w1094, w1093, w1092, w1091, w1090, w1089, w1088, w1087) -> (w1081:bool[])
            n341 = case shown="True" w1085 {
              tunnel: w1086 -> [w1129 w1141]
              tunnel: w1070 -> [w1128 w1140]
              tunnel: [w1127 w1139] -> w1080
              tunnel: [w1126 w1138] -> w1065
              tunnel: w1084 -> [w1125 _]
              tunnel: w1083 -> [w1119 _]
              tunnel: w1082 -> [w1122 w1134]
              tunnel: w1081 -> [w1117 w1133]
              tunnel: w1076 -> [_ _]
              tunnel: w1069 -> [w1116 w1131]
              frame False {
                n342 = local read "SHIFT"() -> (w1124:string)
                n343 = call "PADMINI_SHIFT_DATE.vi"("SHIFT"=w1124) -> ("date/time string"=w1123:string)  [unwired: 10 in]
                n344 = Bundle("SHIFT"=w1124, "date/time string"=w1123, w1122, w1117, w1116) -> (w1115:T15)  [unwired: 1 in]
                n345 = Format Into String(format string="where BARCODE='%s'", w1119) -> (resulting string=w1118:string)  [unwired: 2 in, 1 out]
                n346 = To Variant(anything=w1115) -> ()  [unwired: 1 out]
                n347 = call <vilib>:"DB Tools Update Data.vi"("condition"=w1118, "data"=w1115, "error in (no error)"=w1128, "columns"=string[] ["SHIFT", "DATE", "ST3_REAL_DATA", "ST3_BOOL_DATA", "ST3_RESULT"], "table"=w1125, "connection reference"=w1129) -> ("error out"=w1126:errorcluster, "connection reference out"=w1127:T11)  [unwired: 4 in]
              }
              frame True {
                n348 = local read "SHIFT"() -> (w1136:string)
                n349 = call "PADMINI_SHIFT_DATE.vi"("SHIFT"=w1136) -> ("date/time string"=w1135:string)  [unwired: 10 in]
                n350 = Bundle("SHIFT"=w1136, "date/time string"=w1135, w1134, w1133, w1131) -> (w1130:T15)  [unwired: 1 in]
                n351 = To Variant(anything=w1130) -> ()  [unwired: 1 out]
                n352 = call <vilib>:"DB Tools Insert Data.vi"("data"=w1130, "error in (no error)"=w1140, "columns"=string[] ["SHIFT", "DATE", "ST3_REAL_DATA", "ST3_BOOL_DATA", "ST3_RESULT", "RESULT"], "table"="ST3_REPORT", "connection reference"=w1141) -> ("error out"=w1138:errorcluster, "connection reference out"=w1139:T11)  [unwired: 5 in]
              }
            }
            n353 = call <vilib>:"Simple Error Handler.vi"("type of dialog (OK msg:1)"=w1064, "error in (no error)"=w1065) -> ("error out"=w1066:errorcluster)  [unwired: 3 in, 4 out]
            n354 = call <vilib>:"Clear Errors.vi"("error in (no error)"=w1066) -> ("error out"=w1063:errorcluster)  [unwired: 5 in, 1 out]
            n355 = flat-sequence {
              tunnel: [w1113] -> w1077
              tunnel: w1078 -> [w1113]
              frame #0 {
                n356 = global write "DATA LOG.vi" "DATA LOG RESET 3"(TRUE ("DATA LOG RESET")) -> ()
              }
            }
            n357 = call "PADMINI_AUTO_DATALOG_DONE3.vi"("Enum"=enum16{"Read", "Write"}."Write", "error in (no error)"=w1063, "I/P"=u16 2) -> ("error out"=w1078:errorcluster)  [unwired: 7 in, 1 out]
          }
          frame "DATALOG4" {
            w1160 = 0 ("disabled index (row)")
            w1177 = T12 2 items=["no dialog", "OK message", "continue or stop message", "OK message + warnings", "continue/stop + warnings"] ("type of dialog (OK msg:1)")
            # "ST4_REAL_DATA\nST4_BOOL_DATA\nDATE\nSHIFT"
            # "datalog of st 4"
            n358 = disable-structure shown="Enabled" {
              frame Disabled {
                n359 = call "barcode st4.vi"("Enum"=enum16{"Read", "Write"}."Read") -> ()  [unwired: 9 in, 2 out]
              }
              frame Enabled {
              }
            }
            n360 = local read "STATION-4 2"() -> (w1224:T3)
            n361 = Unbundle By Name(w1224) -> ("BARCODE"=w1184:string, "OK PART"=w1218:dbl, "NOK PART"=w1217:dbl, "TOTAL"=w1216:dbl, "CYCLE TIME"=w1223:dbl, "PARAMETER 1"=w1222:dbl, "PARAMETER 2"=w1221:dbl, "PARAMETER 3"=w1220:dbl, "PARAMETER 4"=w1219:dbl, "SCANNER"=w1215:bool, "CYCLE STATUS"=w1214:bool, "PARAMETER 1"=w1213:bool, "PARAMETER 2"=w1212:bool, "PARAMETER 3"=w1211:bool, "PARAMETER 4"=w1210:bool, "PARAMETER 5"=w1209:bool, "PARAMETER 6"=w1208:bool, "PARAMETER 7"=w1207:bool, "PARAMETER 8"=w1206:bool, "PARAMETER 9"=w1205:bool, "PARAMETER 10"=w1204:bool, "CYCLE RESULT"=w1195:bool)  [unwired: 7 out]
            n362 = call "PADMINI_AUTO_CYCLE STATE4.vi"("Enum"=enum16{"Read", "Write"}."Read", "error in (no error)"=w1180) -> ("error out"=w1170:errorcluster, "Input 2"=w1190:u16[])  [unwired: 8 in]
            n363 = Index Array(array=w1190, index=2) -> (element=w1193:u16)
            n364 = Index Array(array=w1188) -> (element=w1189:string)  [unwired: 1 in]
            n365 = case shown="0" w1193 {
              tunnel: ["" "OK" "NOK" "Aborted"] -> w1192
              frame 0 {
              }
              frame 1, Default {
              }
              frame 2 {
              }
              frame 3 {
              }
            }
            n366 = call <vilib>:"Trim Whitespace.vi"("string"=w1189) -> ("trimmed string"=w1183:string)  [unwired: 1 in]
            n367 = call <vilib>:"Trim Whitespace.vi"("string"=w1184) -> ("trimmed string"=w1182:string)  [unwired: 1 in]
            n368 = call <vilib>:"Clear Errors.vi"("error in (no error)"=w1180) -> ("error out"=w1179:errorcluster)  [unwired: 5 in, 1 out]
            n369 = Build Array(w1218, w1217, w1216, w1223, w1222, w1221, w1220, w1219) -> (w1202:dbl[])
            "LOG DATA 2" <- w1202
            n370 = Build Array(w1215, w1214, w1213, w1212, w1211, w1210, w1209, w1208, w1207, w1206, w1205, w1204) -> (w1201:bool[])
            n371 = Delete From Array(array=w1188, length=1, index=0) -> (array with subset deleted=w1185:string[])  [unwired: 1 out]
            n372 = disable-structure shown="Enabled" {
              disable-tunnel: w1183 -> [w1230 _]
              disable-tunnel: w1182 -> [w1229 _]
              disable-tunnel: [w1228 w1235] -> w1166
              disable-tunnel: w1179 -> [_ w1234]
              disable-tunnel: [_ w1233] -> w1181
              frame Disabled {
                n373 = Empty String/Path?(string/path=w1230) -> (empty?=w1231:bool)
                n374 = Select(t=w1229, s=w1231, f=w1230) -> (s? t:f=w1228:string)
              }
              frame Enabled {
                n375 = call "REAS BARCODE STRING.vi"("error in (no error)"=w1234, "Enum"=enum16{"Read", "Write"}."Read") -> ("error out"=w1233:errorcluster, "Input 2"=w1235:string)  [unwired: 8 in]
                "Input 3" <- w1235
              }
            }
            n376 = Format Into String(format string="where BARCODE='%s'", w1166) -> (resulting string=w1165:string)  [unwired: 2 in, 1 out]
            n377 = call <vilib>:"DB Tools Select Data.vi"("condition"=w1165, "error in (no error)"=w1170, "columns"=string[] ["SHIFT", "DATE", "ST4_REAL_DATA", "ST4_BOOL_DATA", "ST4_RESULT"], "table"=w1164, "connection reference"=w1169) -> ("error out"=w1173:errorcluster, "data"=w1172:variant[][], "connection reference out"=w1168:T11)  [unwired: 1 in]
            n378 = Variant To Data(error in=w1173, type=string[][] [], Variant=w1172) -> (data=w1162:string[][], error out=w1147:errorcluster)
            n379 = Index Array(array=w1162, index (row) #1=w1160, index (col) #1=2 ("disabled index (col)"), index (row) #2=w1160, index (col) #2=3 ("disabled index (col)"), index (row) #3=w1160, index (col) #3=4 ("disabled index (col)")) -> (element #1=w1150:string, element #3=w1157:string)  [unwired: 1 out]
            n380 = Unflatten From String(type=dbl[] [] ("subarray"), binary string=w1150, error in (no error)=w1147) -> (value=w1153:dbl[], error out=w1155:errorcluster)  [unwired: 2 in, 1 out]
            n381 = call <vilib>:"Clear Errors.vi"("error in (no error)"=w1155) -> ("error out"=w1146:errorcluster)  [unwired: 5 in, 1 out]
            n382 = Delete From Array(array=w1153, length=3, index=0) -> (array with subset deleted=w1149:dbl[])  [unwired: 1 out]
            "array w/ subset deleted" <- w1149
            n383 = Equal?(x=w1157, y="OK") -> (x = y?=w1144:bool)
            n384 = Search 1D Array(1D array=w1149, element=0.0) -> (index of element=w1145:i32)  [unwired: 1 in]
            n385 = case shown="-1" w1145 {
              tunnel: [FALSE TRUE] -> w1143
              frame 0, Default {
              }
              frame -1 {
              }
            }
            n386 = And(x=w1144, y=w1143) -> (x .and. y?=w1142:bool)
            n387 = case shown="False" w1203 {
              tunnel: w1168 -> [w1260 w1282]
              tunnel: w1146 -> [_ w1281]
              tunnel: [w1259 w1280] -> w1200
              tunnel: [w1258 w1279] -> w1176
              tunnel: w1164 -> [w1257 _]
              tunnel: w1166 -> [w1247 _]
              tunnel: w1202 -> [w1254 w1275]
              tunnel: w1201 -> [w1250 w1274]
              tunnel: w1195 -> [_ _]
              tunnel: w1192 -> [w1249 w1272]
              tunnel: w1181 -> [w1245 _]
              tunnel: w1142 -> [w1244 _]
              frame False {
                n388 = local read "SHIFT"() -> (w1256:string)
                n389 = call <vilib>:"Trim Whitespace.vi"("string"=w1247) -> ("trimmed string"=w1246:string)  [unwired: 1 in]
                "LOG DATA" <- w1246
                n390 = call "PADMINI_SHIFT_DATE.vi"("SHIFT"=w1256) -> ("date/time string"=w1255:string)  [unwired: 10 in]
                n391 = Bundle("SHIFT"=w1256, "date/time string"=w1255, w1254, w1250, w1249) -> (w1248:T15)  [unwired: 1 in]
                n392 = To Variant(anything=w1248) -> ()  [unwired: 1 out]
                n393 = Format Into String(format string="where BARCODE='%s'", w1246) -> (resulting string=w1251:string)  [unwired: 2 in, 1 out]
                "resulting string" <- w1251
                n394 = case shown="False" w1244 {
                  tunnel: w1260 -> [w1268 w1269]
                  tunnel: [w1267 w1269] -> w1259
                  tunnel: [w1266 w1270] -> w1258
                  tunnel: w1257 -> [w1265 _]
                  tunnel: string[] ["SHIFT", "DATE", "ST4_REAL_DATA", "ST4_BOOL_DATA", "ST4_RESULT"] -> [w1264 _]
                  tunnel: w1251 -> [w1263 _]
                  tunnel: w1248 -> [w1262 _]
                  tunnel: w1245 -> [w1261 w1270]
                  frame False {
                    n395 = call <vilib>:"DB Tools Update Data.vi"("condition"=w1263, "data"=w1262, "error in (no error)"=w1261, "columns"=w1264, "table"=w1265, "connection reference"=w1268) -> ("error out"=w1266:errorcluster, "connection reference out"=w1267:T11)  [unwired: 4 in]
                  }
                  frame True {
                  }
                }
                "error out 5" <- w1258
              }
              frame True {
                n396 = local read "SHIFT"() -> (w1277:string)
                n397 = call "PADMINI_SHIFT_DATE.vi"("SHIFT"=w1277) -> ("date/time string"=w1276:string)  [unwired: 10 in]
                n398 = Bundle("SHIFT"=w1277, "date/time string"=w1276, w1275, w1274, w1272) -> (w1271:T15)  [unwired: 1 in]
                n399 = To Variant(anything=w1271) -> ()  [unwired: 1 out]
                n400 = call <vilib>:"DB Tools Insert Data.vi"("data"=w1271, "error in (no error)"=w1281, "columns"=string[] ["SHIFT", "DATE", "ST4_REAL_DATA", "ST4_BOOL_DATA", "ST4_RESULT", "RESULT"], "table"="ST4_REPORT", "connection reference"=w1282) -> ("error out"=w1279:errorcluster, "connection reference out"=w1280:T11)  [unwired: 5 in]
              }
            }
            n401 = call <vilib>:"Simple Error Handler.vi"("type of dialog (OK msg:1)"=w1177, "error in (no error)"=w1176) -> ("error out"=w1178:errorcluster)  [unwired: 3 in, 4 out]
            n402 = call <vilib>:"Clear Errors.vi"("error in (no error)"=w1178) -> ("error out"=w1175:errorcluster)  [unwired: 5 in, 1 out]
            n403 = flat-sequence {
              tunnel: [w1242] -> w1196
              tunnel: w1197 -> [w1242]
              frame #0 {
                n404 = global write "DATA LOG.vi" "DATA LOG RESET 4"(TRUE ("DATA LOG RESET")) -> ()
                n405 = local write "DATA"(FALSE ("Boolean 6")) -> ()
              }
            }
            n406 = call "PADMINI_AUTO_DATALOG_DONE4.vi"("Enum"=enum16{"Read", "Write"}."Write", "error in (no error)"=w1175, "I/P"=u16 2) -> ("error out"=w1197:errorcluster)  [unwired: 7 in, 1 out]
          }
          frame "BARCODE RECIPE" {
            w1289 = string[][] []
            w1299 = string[] ["BARCODE_RECIPE"] ("columns")
            w1292 = "BARCODE_RECIPE" ("table")
            # "NOT USED THIS CASE  AFTER TAHT LOGIC IS CHANGE  BARCODE RECIPE LOAD IN SETTING WINDOW"
            n407 = local read "BARCODE RECIPE"() -> (w1300:string)
            n408 = Format Into String(format string="WHERE BARCODE_RECIPE = '%s' ", w1300) -> (resulting string=w1298:string)  [unwired: 2 in, 1 out]
            n409 = call <vilib>:"DB Tools Select Data.vi"("condition"=w1298, "error in (no error)"=w1307, "columns"=w1299, "table"=w1292, "connection reference"=w1308) -> ("error out"=w1304:errorcluster, "data"=w1305:variant[][], "connection reference out"=w1301:T11)  [unwired: 1 in]
            n410 = Variant To Data(error in=w1304, type=w1289, Variant=w1305) -> (data=w1295:string[][], error out=w1302:errorcluster)
            n411 = Empty Array?(array=w1295) -> (empty?=w1303:bool)
            n412 = case shown="False" w1303 {
              tunnel: w1302 -> [w1309 w1318]
              tunnel: w1301 -> [w1310 w1317]
              tunnel: [w1310 w1316] -> w1293
              tunnel: [w1309 w1315] -> w1291
              tunnel: w1300 -> [_ w1314]
              tunnel: w1292 -> [_ w1312]
              tunnel: w1299 -> [_ w1311]
              tunnel: w1298 -> [_ _]
              frame False {
              }
              frame True {
                n413 = Bundle("BARCODE RECIPE"=w1314) -> (w1313:cluster{" BARCODE RECIPE":string})  [unwired: 1 in]
                n414 = call <vilib>:"DB Tools Insert Data.vi"("data"=w1313, "error in (no error)"=w1318, "columns"=w1311, "table"=w1312, "connection reference"=w1317) -> ("error out"=w1315:errorcluster, "connection reference out"=w1316:T11)  [unwired: 5 in]
              }
            }
            n415 = call <vilib>:"DB Tools Select Data.vi"("error in (no error)"=w1291, "table"=w1292, "connection reference"=w1293) -> ("error out"=w1286:errorcluster, "data"=w1288:variant[][], "connection reference out"=w1290:T11)  [unwired: 3 in]
            n416 = Variant To Data(error in=w1286, type=w1289, Variant=w1288) -> (data=w1287:string[][], error out=w1285:errorcluster)
            n417 = Index Array(array=w1287, index (col)=0 ("disabled index (col)")) -> (element=w1294:string[])  [unwired: 1 in]
            n418 = property on="BARCODE RECIPE" class="CmbBox"("Strings[]"=w1294) -> ()  [unwired: 2 in, 2 out]
          }
          frame "EMERGENCY STOP" {
          }
          frame "STOP" {
            n419 = global read "Global 1.vi" "BARCODE RECIPE"() -> (w1327:string)
            n420 = Bundle("BARCODE RECIPE"=w1327) -> (w1326:cluster{"BARCODE RECIPE":string})  [unwired: 1 in]
            n421 = call <vilib>:"DB Tools Update Data.vi"("data"=w1326, "error in (no error)"=w1332, "columns"=string[] ["PREVIOUS_LOADED_RECIPE"], "table"="BARCODE_RECIPE", "connection reference"=w1330) -> ("error out"=w1331:errorcluster, "connection reference out"=w1329:T11)  [unwired: 5 in]
          }
        }
      }
      frame Error {
        # "Return true in any case that should stop the loop."
      }
    }
    n422 = Wait (ms)(milliseconds to wait=u32 100) -> ()  [unwired: 1 out]
  }
  n423 = while {
    shift-right: [w1409] -> w102
    shift-left: w19 -> [w1341]
    shift-right: [w1410] -> w96
    shift-left: w100 -> [w1418]
    stop <- w1408 stop-if-true
    w1406 = enum16{"Read", "Write"}."Read" ("Enum")
    # "ST 4 Cycle start bit"
    # "ST 3 Cycle start bit"
    # "ST 2 Cycle start bit"
    # "Barcode Scan Data"
    # "Data Lock"
    n424 = global read "Global 1.vi" "PLC COMM"() -> (→"PLC COM.":bool)
    n425 = global read "Global 1.vi" "PLC 1"() -> (→"Boolean":bool)
    n426 = global read "Global 1.vi" "PLC 2"() -> (→"Boolean 2":bool)
    n427 = global read "Global 1.vi" "PLC 3"() -> (→"Boolean 3":bool)
    n428 = global read "Global 1.vi" "PLC 4"() -> (→"Boolean 4":bool)
    n429 = call <vilib>:"Clear Errors.vi"("error in (no error)"=w1341) -> ("error out"=w1340:errorcluster)  [unwired: 5 in, 1 out]
    n430 = call "READ EMERGENCY BIT.vi"("Enum"=enum16{"Read", "Write"}."Read", "error in (no error)"=w1340) -> ("Array Out"=w1347:dbl[])  [unwired: 8 in, 1 out]
    n431 = call "PADMINI_AUTO_CYCLE STATE2.vi"("Enum"=enum16{"Read", "Write"}."Read", "error in (no error)"=w1340) -> ("Input 2"=w1377:u16[])  [unwired: 8 in, 1 out]
    n432 = call "PADMINI_AUTO_CYCLE STATE3.vi"("Enum"=enum16{"Read", "Write"}."Read", "error in (no error)"=w1340) -> ("Input 2"=w1372:u16[])  [unwired: 8 in, 1 out]
    n433 = call "PADMINI_AUTO_CYCLE_BIT.vi"("Enum"=w1406, "error in (no error)"=w1340) -> ("Input 2"=w1405:u16[])  [unwired: 8 in, 1 out]
    n434 = call "PADMINI_AUTO_CYCLE_BIT2.vi"("Enum"=w1406, "error in (no error)"=w1340) -> ("Input 2"=w1402:u16[])  [unwired: 8 in, 1 out]
    n435 = call "PADMINI_AUTO_CYCLE_BIT3.vi"("Enum"=w1406, "error in (no error)"=w1340) -> ("Input 2"=w1400:u16[])  [unwired: 8 in, 1 out]
    n436 = call "PADMINI_AUTO_CYCLE_BIT4.vi"("Enum"=w1406, "error in (no error)"=w1340) -> ("Input 2"=w1401:u16[])  [unwired: 8 in, 1 out]
    n437 = call "PADMINI_AUTO_CYCLE STATE4.vi"("Enum"=enum16{"Read", "Write"}."Read", "error in (no error)"=w1340) -> ("Input 2"=w1368:u16[])  [unwired: 8 in, 1 out]
    n438 = Index Array(array=w1368, index=0) -> (element=w1367:u16)
    n439 = Index Array(array=w1372, index=0) -> (element=w1371:u16)
    n440 = Index Array(array=w1347) -> (element=w1346:dbl)  [unwired: 1 in]
    n441 = Index Array(array=w1377, index=0) -> (element=w1375:u16)
    n442 = Index Array(array=w1400, index #1=2 ("index"), index #2=1 ("index")) -> (element #2=w1383:u16)  [unwired: 1 out]
    n443 = Index Array(array=w1401, index #1=2 ("index"), index #2=1 ("index")) -> (element #2=w1343:u16)  [unwired: 1 out]
    n444 = Index Array(array=w1405, index #1=2 ("index"), index #2=1 ("index")) -> (element #1=w1393:u16, element #2=w1392:u16, element #3=w1379:u16)  [unwired: 1 in]
    n445 = Index Array(array=w1402, index #1=2 ("index"), index #2=1 ("index")) -> (element #2=w1391:u16)  [unwired: 1 out]
    n446 = global read "DATA LOG.vi" "op 40"() -> (w1364:i32)
    n447 = global read "DATA LOG.vi" "op 60"() -> (w1363:i32)
    n448 = global read "DATA LOG.vi" "op 30"() -> (w1365:i32)
    n449 = call "ST4 DATALOG.vi"("Numeric"=w1343) -> ("Boolean"=w1342:bool)  [unwired: 9 in, 1 out]
    "Boolean 6" <- w1342
    n450 = call "VALUE_CHANGE1.vi"("Numeric"=w1393) -> ("Boolean"=w1382:bool)  [unwired: 9 in, 1 out]
    n451 = call "VALUE_CHANGE - ST1_RESULT.vi"("Numeric"=w1392) -> ("Boolean"=w1356:bool)  [unwired: 9 in, 1 out]
    n452 = call "VALUE_CHANGE2.vi"("Numeric"=w1365) -> ("Boolean"=w1366:bool)  [unwired: 9 in, 1 out]
    n453 = call "VALUE_CHANGE - ST2_RESULT.vi"("Numeric"=w1391) -> ("Boolean"=w1390:bool)  [unwired: 9 in, 1 out]
    n454 = call "VALUE_CHANGE3.vi"("Numeric"=w1364) -> ("Boolean"=w1358:bool)  [unwired: 9 in, 1 out]
    n455 = call "VALUE_CHANGE - ST3_RESULT.vi"("Numeric"=w1383) -> ("Boolean"=w1389:bool)  [unwired: 9 in, 1 out]
    n456 = call "VALUE_CHANGE4.vi"("Numeric"=w1363) -> ("Boolean"=w1388:bool)  [unwired: 9 in, 1 out]
    n457 = call "VALUE_CHANGE - ST1_RESULT.vi"("Numeric"=w1379) -> ("Boolean"=w1381:bool)  [unwired: 9 in, 1 out]
    n458 = call "VALUE_CHANGE - ST1_RESULT.vi"("Numeric"=w1375) -> ("Boolean"=w1380:bool)  [unwired: 9 in, 1 out]
    n459 = call "VALUE_CHANGE - ST1_RESULT.vi"("Numeric"=w1371) -> ("Boolean"=w1362:bool)  [unwired: 9 in, 1 out]
    n460 = call "VALUE_CHANGE - ST1_RESULT.vi"("Numeric"=w1367) -> ("Boolean"=w1360:bool)  [unwired: 9 in, 1 out]
    n461 = call "VALUE_CHANGE - ST1_RESULT.vi"("Numeric"=w1346) -> ("Boolean"=w1344:bool)  [unwired: 9 in, 1 out]
    n462 = call <userlib>:"Boolean Trigger__ogtk.vi"("Boolean Input"=w1356) -> ("Rising Edge"=w1355:bool)  [unwired: 1 in, 1 out]
    n463 = call <userlib>:"Boolean Trigger__ogtk.vi"("Boolean Input"=w1358) -> ("Rising Edge"=w1357:bool)  [unwired: 1 in, 1 out]
    n464 = call "FIND TURE FOR AUTO.vi"("CYCLE START"="NEXT") -> ("Boolean"=w1352:bool)  [unwired: 8 in]
    n465 = call "FIND TURE FOR AUTO.vi"("CYCLE START"="Back") -> ("Boolean"=w1351:bool)  [unwired: 8 in]
    n466 = call <userlib>:"Boolean Trigger__ogtk.vi"("Boolean Input"=w1344) -> ("Rising Edge"=w1345:bool)  [unwired: 1 in, 1 out]
    n467 = call "FIND TURE FOR AUTO.vi"("CYCLE START"="Add Button") -> ("Boolean"=w1349:bool)  [unwired: 8 in]
    n468 = call <userlib>:"Boolean Trigger__ogtk.vi"("Boolean Input"=w1362) -> ("Rising Edge"=w1361:bool)  [unwired: 1 in, 1 out]
    n469 = call <userlib>:"Boolean Trigger__ogtk.vi"("Boolean Input"=w1360) -> ("Rising Edge"=w1359:bool)  [unwired: 1 in, 1 out]
    n470 = global write "Global 1.vi" "EMERGENCY STOP"(w1344) -> ()
    n471 = Build Array(w1382, w1355, w1366, w1390, w1357, w1389, w1388, w1342, w1381, w1380, w1361, w1359, w1352, w1351, w1349, w1345) -> (w1407:bool[])
    n472 = local read "Shift_change"() -> (w1416:bool)
    n473 = for {
      tunnel: w1407 -> [w1583] mode=indexing
      tunnel: [w1584] -> w1419 mode=indexing if=w1583
      i -> [w1584]
    }
    n474 = case shown="True" w1416 {
      tunnel: w1340 -> [w1435 w1448]
      tunnel: [w1436 w1447] -> w1415
      frame False {
        n475 = local read "SHIFT_DATA 2"() -> (w1438:string[])
        n476 = call "String To Time_4.vi"("error in (no error)"=w1435, "String Array In"=w1438) -> ("error out"=w1434:errorcluster, "Time Stamp Out"=w1433:timestamp[])  [unwired: 8 in]
        "Time Stamp Out 4" <- w1433
        n477 = Get Date/Time In Seconds() -> (seconds since 1Jan1904=w1437:timestamp)
        n478 = call "Shift Calculation_4.vi"("error in (no error)"=w1434, "Current Time"=w1437, "Time Stamp Out"=w1433) -> ("error out"=w1432:errorcluster, "Shift"=w1431:i32)  [unwired: 7 in]
        n479 = call <vilib>:"Clear Errors.vi"("error in (no error)"=w1432) -> ()  [unwired: 5 in, 2 out]
        n480 = case shown="4" w1431 {
          tunnel: ["A" "B" "C" "D"] -> w1436
          frame 1, Default {
          }
          frame 2 {
          }
          frame 3 {
          }
          frame 4 {
          }
        }
      }
      frame True {
        n481 = local read "SHIFT_DATA"() -> (w1446:string[])
        n482 = call "String To Time.vi"("error in (no error)"=w1448, "String Array In"=w1446) -> ("error out"=w1445:errorcluster, "Time Stamp Out"=w1450:timestamp[])  [unwired: 8 in]
        "Time Stamp Out" <- w1450
        n483 = Get Date/Time In Seconds() -> (seconds since 1Jan1904=w1449:timestamp)
        n484 = call "Shift Calculation.vi"("error in (no error)"=w1445, "Current Time"=w1449, "Time Stamp Out"=w1450) -> ("error out"=w1444:errorcluster, "Shift"=w1443:i32)  [unwired: 7 in]
        "Shift 4" <- w1443
        n485 = call <vilib>:"Clear Errors.vi"("error in (no error)"=w1444) -> ()  [unwired: 5 in, 2 out]
        n486 = case shown="3" w1443 {
          tunnel: ["A" "B" "C"] -> w1447
          frame 1, Default {
          }
          frame 2 {
          }
          frame 3 {
          }
        }
      }
    }
    "SHIFT" <- w1415
    n487 = for {
      tunnel: w1419 -> [w1454] mode=indexing
      shift-right: [w1458] -> w1412
      shift-left: w1418 -> [w1457]
      shift-right: [w1456] -> w1411
      shift-left: w1340 -> [w1455]
      n488 = case shown="8" w1454 {
        tunnel: [w1460 w1466 w1472 w1480 w1486 w1494 w1500 w1508 w1515 w1522 w1529 w1540 w1552 w1569 w1572 w1576 w1581] -> w1458
        tunnel: w1457 -> [w1462 w1468 w1474 w1482 w1488 w1496 w1502 w1510 w1517 w1524 w1530 w1541 w1553 w1569 w1572 w1573 w1578]
        tunnel: [w1459 w1465 w1471 w1479 w1485 w1493 w1499 w1507 w1514 w1521 w1528 w1539 w1551 w1568 w1571 w1575 w1580] -> w1456
        tunnel: w1455 -> [w1461 w1467 w1473 w1481 w1487 w1495 w1501 w1509 w1516 w1523 w1526 w1537 w1549 w1568 w1571 w1574 w1579]
        frame -1, Default {
          # "DEFAULT"
          n489 = Enqueue Element(queue=w1462, element=cluster{"CASE":T9} {"CASE"=enum."-1"}, error in (no error)=w1461) -> (queue out=w1460:refnum<queue>, error out=w1459:errorcluster)  [unwired: 1 in, 1 out]
        }
        frame 0 {
          # "SCAN BARCODE 1"
          n490 = Enqueue Element(queue=w1468, element=cluster{"CASE":T9} {"CASE"=enum."SCAN1"}, error in (no error)=w1467) -> (queue out=w1466:refnum<queue>, error out=w1465:errorcluster)  [unwired: 1 in, 1 out]
        }
        frame 1 {
          # "DATALOG OF ST 1"
          n491 = disable-structure shown="Enabled" {
            disable-tunnel: [w1475 w1476] -> w1469
            frame Enabled {
              n492 = local read "OP 10 & OP 21"() -> (w1475:T2)
            }
            frame Disabled {
              n493 = local read "OP 10 & OP 20"() -> (w1476:T6)
            }
          }
          "STATION-1 2" <- w1469
          n494 = Enqueue Element(queue=w1474, element=cluster{"CASE":T9} {"CASE"=enum."DATALOG1"}, error in (no error)=w1473) -> (queue out=w1472:refnum<queue>, error out=w1471:errorcluster)  [unwired: 1 in, 1 out]
        }
        frame 2 {
          # "SCAN BARCODE FOR ST 2"
          n495 = global write "DATA LOG.vi" "op 30"(0 ("op 30")) -> ()
          n496 = Enqueue Element(queue=w1482, element=cluster{"CASE":T9} {"CASE"=enum."SCAN2"}, error in (no error)=w1481) -> (queue out=w1480:refnum<queue>, error out=w1479:errorcluster)  [unwired: 1 in, 1 out]
        }
        frame 3 {
          # "DATALOG OF ST 2"
          n497 = disable-structure shown="Enabled" {
            disable-tunnel: [w1489 w1490] -> w1483
            frame Disabled {
              n498 = local read "OP 30"() -> (w1489:T5)
            }
            frame Enabled {
              n499 = local read "OP 30"() -> (w1490:T5)
            }
          }
          "STATION-2 2" <- w1483
          n500 = Enqueue Element(queue=w1488, element=cluster{"CASE":T9} {"CASE"=enum."DATALOG2"}, error in (no error)=w1487) -> (queue out=w1486:refnum<queue>, error out=w1485:errorcluster)  [unwired: 1 in, 1 out]
        }
        frame 4 {
          # "SCAN BARCODE FOR ST 3"
          n501 = global write "DATA LOG.vi" "op 40"(0 ("op 30")) -> ()
          n502 = Enqueue Element(queue=w1496, element=cluster{"CASE":T9} {"CASE"=enum."SCAN3"}, error in (no error)=w1495) -> (queue out=w1494:refnum<queue>, error out=w1493:errorcluster)  [unwired: 1 in, 1 out]
        }
        frame 5 {
          # "DATALOG OF ST 3"
          n503 = disable-structure shown="Enabled" {
            disable-tunnel: [w1503 w1504] -> w1497
            frame Disabled {
              n504 = local read "OP 40"() -> (w1503:T7)
            }
            frame Enabled {
              n505 = local read "OP 40"() -> (w1504:T7)
            }
          }
          "STATION-3 2" <- w1497
          n506 = Enqueue Element(queue=w1502, element=cluster{"CASE":T9} {"CASE"=enum."DATALOG3"}, error in (no error)=w1501) -> (queue out=w1500:refnum<queue>, error out=w1499:errorcluster)  [unwired: 1 in, 1 out]
        }
        frame 6 {
          # "SCAN BARCODE FOR ST 4"
          n507 = global write "DATA LOG.vi" "op 60"(0 ("op 30")) -> ()
          n508 = Enqueue Element(queue=w1510, element=cluster{"CASE":T9} {"CASE"=enum."SCAN4"}, error in (no error)=w1509) -> (queue out=w1508:refnum<queue>, error out=w1507:errorcluster)  [unwired: 1 in, 1 out]
        }
        frame 7 {
          # "DATALOG OF ST 4"
          n509 = disable-structure shown="Enabled" {
            disable-tunnel: [w1518 w1519] -> w1512
            frame Enabled {
              n510 = local read "OP 61"() -> (w1518:T1)
            }
            frame Disabled {
              n511 = local read "OP 60"() -> (w1519:T8)
            }
          }
          "STATION-4 2" <- w1512
          n512 = Enqueue Element(queue=w1517, element=cluster{"CASE":T9} {"CASE"=enum."DATALOG4"}, error in (no error)=w1516) -> (queue out=w1515:refnum<queue>, error out=w1514:errorcluster)  [unwired: 1 in, 1 out]
          "DATA" <- TRUE
        }
        frame 8 {
          # "DATALOG OF ST 4"
          n513 = Enqueue Element(queue=w1524, element=cluster{"CASE":T9} {"CASE"=enum."-1"}, error in (no error)=w1523) -> (queue out=w1522:refnum<queue>, error out=w1521:errorcluster)  [unwired: 1 in, 1 out]
        }
        frame 9 {
          # "FOR ST 2 : ON CYCLE START BIT WRITE BARCODE STATUS '0' TO PLC"
          n514 = flat-sequence {
            tunnel: [w1532] -> w1525
            tunnel: w1526 -> [w1533]
            frame #0 {
              n515 = global write "DATA LOG.vi" "OP30 ST 2 STRING"("" ("OP30 ST 2 STRING")) -> ()
              n516 = call "PADMINI_AUTO_BARCODE_STATUS2.vi"("Enum"=enum16{"Read", "Write"}."Write", "error in (no error)"=w1533, "I/P"=u16 0) -> ("error out"=w1532:errorcluster)  [unwired: 7 in, 1 out]
            }
          }
          n517 = Enqueue Element(queue=w1530, element=cluster{"CASE":T9} {"CASE"=enum."-1"}, error in (no error)=w1525) -> (queue out=w1529:refnum<queue>, error out=w1528:errorcluster)  [unwired: 1 in, 1 out]
        }
        frame 10 {
          # "FOR ST 3 : ON CYCLE START BIT WRITE BARCODE STATUS '0' TO PLC"
          n518 = flat-sequence {
            tunnel: [w1546] -> w1536
            tunnel: w1537 -> [w1547]
            frame #0 {
              n519 = global write "DATA LOG.vi" "ST 3 STRING 2"("" ("OP30 ST 2 STRING")) -> ()
              n520 = global write "DATA LOG.vi" "scan op 40"(TRUE ("scan op 40")) -> ()
              n521 = call "PADMINI_AUTO_BARCODE_STATUS3.vi"("Enum"=enum16{"Read", "Write"}."Write", "error in (no error)"=w1547, "I/P"=u16 0) -> ("error out"=w1546:errorcluster)  [unwired: 7 in, 1 out]
            }
          }
          n522 = Enqueue Element(queue=w1541, element=cluster{"CASE":T9} {"CASE"=enum."-1"}, error in (no error)=w1536) -> (queue out=w1540:refnum<queue>, error out=w1539:errorcluster)  [unwired: 1 in, 1 out]
        }
        frame 11 {
          # "FOR ST 4 : ON CYCLE START BIT WRITE BARCODE STATUS '0' TO PLC"
          n523 = flat-sequence {
            tunnel: w1549 -> [w1555]
            tunnel: [w1554] -> w1548
            frame #0 {
              n524 = disable-structure shown="Enabled" {
                disable-tunnel: w1555 -> [w1559 w1563]
                disable-tunnel: [w1557 w1565] -> w1554
                frame Disabled {
                  n525 = global write "DATA LOG.vi" "scan op 60"(TRUE ("scan op 60")) -> ()
                  n526 = global write "DATA LOG.vi" "ST 4 STRING 3"("") -> ()
                  n527 = call "PADMINI_AUTO_BARCODE_STATUS4.vi"("Enum"=enum16{"Read", "Write"}."Write", "error in (no error)"=w1559, "I/P"=u16 0) -> ("error out"=w1557:errorcluster)  [unwired: 7 in, 1 out]
                }
                frame Enabled {
                  n528 = call <vilib>:"Clear Errors.vi"("error in (no error)"=w1563) -> ("error out"=w1562:errorcluster)  [unwired: 5 in, 1 out]
                  n529 = call "PADMINI_AUTO_BARCODE_STATUS4.vi"("Enum"=enum16{"Read", "Write"}."Write", "error in (no error)"=w1562, "I/P"=u16 0) -> ("error out"=w1565:errorcluster)  [unwired: 7 in, 1 out]
                }
              }
            }
          }
          n530 = Enqueue Element(queue=w1553, element=cluster{"CASE":T9} {"CASE"=enum."-1"}, error in (no error)=w1548) -> (queue out=w1552:refnum<queue>, error out=w1551:errorcluster)  [unwired: 1 in, 1 out]
        }
        frame 12 {
          n531 = property on="Tab Control" class="TabCtl (strict)"("Value"=enum32{"Page 1", "Page 2"}."Page 2" ("Tab Control")) -> ()  [unwired: 2 in, 2 out]
        }
        frame 13 {
          n532 = property on="Tab Control" class="TabCtl (strict)"("Value"=enum32{"Page 1", "Page 2"}."Page 1" ("Tab Control")) -> ()  [unwired: 2 in, 2 out]
        }
        frame 14 {
          n533 = Enqueue Element(queue=w1573, element=cluster{"CASE":T9} {"CASE"=enum."BARCODE RECIPE"}, error in (no error)=w1574) -> (queue out=w1576:refnum<queue>, error out=w1575:errorcluster)  [unwired: 1 in, 1 out]
        }
        frame 15 {
          n534 = Enqueue Element(queue=w1578, element=cluster{"CASE":T9} {"CASE"=enum."EMERGENCY STOP"}, error in (no error)=w1579) -> (queue out=w1581:refnum<queue>, error out=w1580:errorcluster)  [unwired: 1 in, 1 out]
        }
      }
    }
    n535 = case shown="True" "stop 2" {
      tunnel: w1412 -> [w1422 w1428]
      tunnel: [w1422 w1427] -> w1410
      tunnel: w1411 -> [w1421 w1426]
      tunnel: [w1421 w1425] -> w1409
      tunnel: [FALSE TRUE] -> w1408
      frame False {
      }
      frame True {
        n536 = Flush Queue(queue=w1428, error in (no error)=w1426) -> (queue out=w1430:refnum<queue>, error out=w1429:errorcluster)  [unwired: 1 out]
        n537 = Enqueue Element(queue=w1430, element=cluster{"CASE":T9} {"CASE"=enum."STOP"}, error in (no error)=w1429) -> (queue out=w1427:refnum<queue>, error out=w1425:errorcluster)  [unwired: 1 in, 1 out]
      }
    }
    "stop" <- w1408
    n538 = Wait (ms)(milliseconds to wait=u32 50) -> ()  [unwired: 1 out]
  }
  n539 = while {
    tunnel: w19 -> [w1601]
    tunnel: w41 -> [w1600]
    tunnel: w39 -> [w1598]
    tunnel: w40 -> [w1597]
    tunnel: w42 -> [w1596]
    tunnel: [w1586] -> w44
    stop <- w1595 stop-if-true
    n540 = flat-sequence {
      tunnel: w1601 -> [w1628]
      tunnel: w1600 -> [w1672]
      tunnel: [w1609] -> w1599
      tunnel: w1598 -> [w1668]
      tunnel: w1597 -> [w1667]
      tunnel: w1596 -> [w1666]
      tunnel: [w1668] -> w1593
      tunnel: [w1667] -> w1591
      tunnel: [w1666] -> w1587
      tunnel: w1599 -> [w1714]
      tunnel: [w1708] -> w1594
      tunnel: w1593 -> [w1733]
      tunnel: [w1732] -> w1592
      tunnel: w1591 -> [w1732]
      tunnel: [w1731] -> w1588
      tunnel: w1587 -> [w1731]
      tunnel: w1594 -> [w1757]
      tunnel: w1592 -> [w1792]
      tunnel: [w1791] -> w1590
      tunnel: [w1790] -> w1589
      tunnel: w1588 -> [w1790]
      tunnel: w1590 -> [w1811]
      tunnel: [w1886] -> w1586
      tunnel: w1589 -> [w1885]
      frame #0 {
        w1650 = 1.0 ("element")
        # "CYCLE STATUS"
        n541 = call "PADMINI_AUTO_BARCODE_STRING.vi"("Enum"=enum16{"Read", "Write"}."Read", "error in (no error)"=w1628) -> ("Input 2"=w1674:string)  [unwired: 8 in, 1 out]
        n542 = call "PADMINI_AUTO_COUNTER_TIME.vi"("Enum"=enum16{"Read", "Write"}."Read", "error in (no error)"=w1628) -> ("Input 2"=w1678:u16[])  [unwired: 8 in, 1 out]
        n543 = call "PADMINI_AUTO_CYCLE_BIT.vi"("Enum"=enum16{"Read", "Write"}."Read", "error in (no error)"=w1628) -> ("Input 2"=w1670:u16[])  [unwired: 8 in, 1 out]
        n544 = property on="OP 10 & OP 21" class="Clust"(error in=w1628) -> (error out=w1608:errorcluster, "Controls[]"=w1627:refnum<vi>[])  [unwired: 1 in, 1 out]
        n545 = call "PADMINI_AUTO_RESULT_DATA.vi"("Enum"=enum16{"Read", "Write"}."Read", "error in (no error)"=w1628) -> ("Input 2"=w1684:dbl[])  [unwired: 8 in, 1 out]
        n546 = property on="OP 10 & OP 20" class="Clust"(error in=w1628) -> (error out=w1619:errorcluster, "Controls[]"=w1618:refnum<vi>[])  [unwired: 1 in, 1 out]
        n547 = call "PADMINI_AUTO_RESULT_DATA_st1_log.vi"("Enum"=enum16{"Read", "Write"}."Read", "error in (no error)"=w1628) -> ("Input 2"=w1643:dbl[])  [unwired: 8 in, 1 out]
        n548 = Index Array(array=w1678) -> (element #1=w1649:u16, element #2=w1677:u16, element #3=w1676:u16, element #4=w1675:u16)  [unwired: 4 in]
        n549 = Index Array(array=w1670) -> (element=w1669:u16)  [unwired: 1 in]
        n550 = Index Array(array=w1684) -> (element #1=w1606:dbl, element #2=w1607:dbl, element #3=w1665:dbl, element #4=w1664:dbl, element #5=w1663:dbl, element #6=w1662:dbl, element #7=w1661:dbl, element #8=w1660:dbl, element #9=w1659:dbl, element #10=w1658:dbl, element #11=w1657:dbl, element #12=w1656:dbl, element #13=w1655:dbl, element #14=w1654:dbl, element #15=w1653:dbl, element #16=w1652:dbl, element #17=w1651:dbl)  [unwired: 17 in]
        n551 = Index Array(array=w1643) -> (element #1=w1641:dbl, element #2=w1640:dbl, element #3=w1639:dbl, element #4=w1638:dbl, element #5=w1637:dbl, element #6=w1636:dbl, element #7=w1635:dbl, element #8=w1634:dbl, element #9=w1633:dbl, element #10=w1632:dbl, element #11=w1631:dbl, element #12=w1630:dbl, element #13=w1629:dbl, element #16=w1611:dbl)  [unwired: 16 in, 2 out]
        n552 = Index Array(array=w1672, index=w1669) -> (element=w1604:string)
        n553 = Array Subset(array=w1618, index=15, length=10) -> (w1617:refnum<vi>[])
        n554 = Array Subset(array=w1627, index=15, length=8) -> (w1624:refnum<vi>[])
        n555 = for {
          shift-right: [w1695] -> w1605
          shift-left: w1608 -> [w1695]
          tunnel: w1624 -> [w1697] mode=indexing
          tunnel: [w1694] -> w1623 mode=indexing
          w1696 = refnum<vi> refnum  # Boolean
          n556 = To More Specific Class(target class=w1696, reference=w1697) -> (specific class reference=w1694:refnum<vi>)  [unwired: 1 in, 1 out]
        }
        n557 = for {
          shift-right: [w1703] -> w1645
          shift-left: w1619 -> [w1703]
          tunnel: w1617 -> [w1705] mode=indexing
          tunnel: [w1702] -> w1689 mode=indexing
          w1704 = refnum<vi> refnum  # Boolean
          n558 = To More Specific Class(target class=w1704, reference=w1705) -> (specific class reference=w1702:refnum<vi>)  [unwired: 1 in, 1 out]
        }
        n559 = Divide(x=w1649, y=10.0) -> (x/y=w1648:dbl)
        n560 = Build Array(w1657, w1656, w1655, w1654, w1653, w1652, w1651, w1650, w1650, w1650) -> (w1683:dbl[])
        n561 = Build Array(w1635, w1634, w1633, w1632, w1631, w1630, w1629) -> (w1620:dbl[])
        n562 = for {
          tunnel: w1689 -> [w1701] mode=indexing
          tunnel: w1683 -> [w1700] mode=indexing
          tunnel: w1645 -> [w1699]
          tunnel: [w1698] -> w1610
          n563 = call "PADMINI_BOOL_COLOR_CHANGE.vi"("error in (no error)"=w1699, "Numeric"=w1700, "Boolean in"=w1701) -> ("error out"=w1698:errorcluster)  [unwired: 8 in]
        }
        n564 = for {
          tunnel: w1623 -> [w1693] mode=indexing
          tunnel: w1620 -> [w1692] mode=indexing
          tunnel: w1605 -> [w1691]
          tunnel: [w1690] -> w1616
          n565 = call "PADMINI_BOOL_COLOR_CHANGE.vi"("error in (no error)"=w1691, "Numeric"=w1692, "Boolean in"=w1693) -> ("error out"=w1690:errorcluster)  [unwired: 8 in]
        }
        "error out" <- w1616
        n566 = control-ref of="CYCLE RESULT"() -> (w1612:refnum<vi>)
        n567 = local read "OP 10 & OP 20"() -> (w1622:T6)
        n568 = Bundle By Name(cluster=w1622, "STATUS"=w1604, "BARCODE"=w1674, "Cycle Time"=w1648, "OK Part"=w1677, "NOK Part"=w1676, "Total"=w1675, "Load at 13.4 mm(N)"=w1606, "Load at 14 mm(N)"=w1607, "Seal Press Load (N)"=w1665, "Spring Height (mm)"=w1664, "Spring and Seal Press Load(N)"=w1663, "Spring & Seal Press Check Load(N)"=w1662, "PARAMETER 7"=w1661, "PARAMETR 8"=w1660, "PARAMETER 9"=w1659, "PARAMETER 10"=w1658) -> (→"OP 10 & OP 20":T6)
        n569 = local read "OP 10 & OP 21"() -> (w1621:T2)
        n570 = Bundle By Name(cluster=w1621, "SPRING LOAD AT 13.4 mm(N)"=w1641, "SPRING LOAD AT 14 mm((N)"=w1640, "SEAL PRESS LOAD(N)"=w1639, "SPRING HEIGHT(mm)"=w1638, "SPRING AND SEAL PRESS LOAD(N)"=w1637, "SPRING AND SEAL PRESS CHECK LOAD(N)"=w1636) -> (→"OP 10 & OP 21":T2)
        n571 = call "PADMINI_AUTO_CYCLE STATE.vi"("Enum"=enum16{"Read", "Write"}."Read", "error in (no error)"=w1610) -> ("error out"=w1609:errorcluster, "Input 2"=w1681:u16[])  [unwired: 8 in]
        n572 = call "PADMINI_RESULT_COLOR_CHANGE .vi"("Numeric"=w1611, "Boolean in"=w1612) -> ()  [unwired: 10 in]
        n573 = control-ref of="Cycle Status"() -> (w1613:refnum<vi>)
        n574 = control-ref of="Cycle Result"() -> (w1615:refnum<vi>)
        n575 = Index Array(array=w1681, index #1=0 ("index")) -> (element #1=w1646:u16, element #3=w1614:u16)  [unwired: 2 in, 1 out]
        n576 = call "PADMINI_STATUS_COLOR_CHANGE .vi"("Numeric"=w1646, "Boolean in"=w1613) -> ()  [unwired: 10 in]
        n577 = call "PADMINI_RESULT_COLOR_CHANGE .vi"("Numeric"=w1614, "Boolean in"=w1615) -> ()  [unwired: 10 in]
      }
      frame #1 {
        n578 = call "PADMINI_AUTO_CYCLE_BIT2.vi"("Enum"=enum16{"Read", "Write"}."Read", "error in (no error)"=w1714) -> ("Input 2"=w1748:u16[])  [unwired: 8 in, 1 out]
        n579 = call "PADMINI_AUTO_BARCODE_STRING2.vi"("Enum"=enum16{"Read", "Write"}."Read", "error in (no error)"=w1714) -> ()  [unwired: 8 in, 2 out]
        n580 = call "PADMINI_AUTO_COUNTER_TIME2.vi"("Enum"=enum16{"Read", "Write"}."Read", "error in (no error)"=w1714) -> ("Input 2"=w1741:u16[])  [unwired: 8 in, 1 out]
        n581 = control-ref of="FORCE (N)"() -> (w1719:refnum<vi>)
        n582 = call "PADMINI_AUTO_RESULT_DATA2.vi"("Enum"=enum16{"Read", "Write"}."Read", "error in (no error)"=w1714) -> ("Input 2"=w1736:dbl[])  [unwired: 8 in, 1 out]
        n583 = Index Array(array=w1741) -> (element #1=w1742:u16, element #2=w1743:u16, element #3=w1744:u16, element #4=w1745:u16)  [unwired: 4 in]
        n584 = Index Array(array=w1748) -> (element=w1749:u16)  [unwired: 1 in]
        n585 = Index Array(array=w1736) -> (element #1=w1730:dbl, element #2=w1729:dbl, element #3=w1728:dbl, element #4=w1727:dbl, element #5=w1726:dbl, element #6=w1725:dbl, element #7=w1724:dbl, element #8=w1723:dbl, element #9=w1722:dbl, element #10=w1721:dbl, element #11=w1717:dbl, element #12=w1716:dbl)  [unwired: 12 in]
        n586 = control-ref of="POSITION (mm)"() -> (w1718:refnum<vi>)
        n587 = Index Array(array=w1733, index=w1749) -> (element=w1750:string)
        n588 = call "PADMINI_BOOL_COLOR_CHANGE.vi"("error in (no error)"=w1714, "Numeric"=w1717, "Boolean in"=w1719) -> ("error out"=w1715:errorcluster)  [unwired: 8 in]
        n589 = Divide(x=w1742, y=u16 10) -> (x/y=w1707:dbl)
        n590 = call "PADMINI_BOOL_COLOR_CHANGE.vi"("error in (no error)"=w1715, "Numeric"=w1716, "Boolean in"=w1718) -> ("error out"=w1711:errorcluster)  [unwired: 8 in]
        n591 = local read "OP 30"() -> (w1734:T5)
        n592 = call "PADMINI_AUTO_CYCLE STATE2.vi"("Enum"=enum16{"Read", "Write"}."Read", "error in (no error)"=w1711) -> ("error out"=w1708:errorcluster, "Input 2"=w1738:u16[])  [unwired: 8 in]
        n593 = Bundle By Name(cluster=w1734, "STATUS"=w1750, "Cycle Time"=w1707, "OK Part"=w1743, "NOK Part"=w1744, "Total"=w1745, "Force (KgF)"=w1730, "POSITION (mm)"=w1729, "PARAMETER 3"=w1728, "PARAMETER 4"=w1727, "PARAMETER 5"=w1726, "PARAMETER 6"=w1725, "PARAMETER 7"=w1724, "PARAMETER 8"=w1723, "PARAMETER 9"=w1722, "PARAMETER 10"=w1721) -> (→"OP 30":T5)
        n594 = Index Array(array=w1738, index #1=0 ("index")) -> (element #1=w1713:u16, element #3=w1710:u16)  [unwired: 2 in, 1 out]
        n595 = control-ref of="Cycle Status"() -> (w1712:refnum<vi>)
        n596 = control-ref of="Cycle Result"() -> (w1709:refnum<vi>)
        n597 = call "PADMINI_STATUS_COLOR_CHANGE .vi"("Numeric"=w1713, "Boolean in"=w1712) -> ()  [unwired: 10 in]
        n598 = call "PADMINI_RESULT_COLOR_CHANGE .vi"("Numeric"=w1710, "Boolean in"=w1709) -> ()  [unwired: 10 in]
      }
      frame #2 {
        n599 = call "PADMINI_AUTO_RESULT_DATA3.vi"("Enum"=enum16{"Read", "Write"}."Read", "error in (no error)"=w1757) -> ("Input 2"=w1807:dbl[])  [unwired: 8 in, 1 out]
        n600 = Index Array(array=w1807) -> (element #1=w1789:dbl, element #2=w1788:dbl, element #3=w1754:dbl, element #4=w1787:dbl, element #5=w1786:dbl, element #6=w1785:dbl, element #7=w1784:dbl, element #8=w1783:dbl, element #9=w1782:dbl, element #10=w1781:dbl, element #11=w1769:dbl, element #12=w1768:dbl, element #13=w1767:dbl, element #14=w1766:dbl, element #15=w1765:dbl, element #16=w1764:dbl, element #17=w1763:dbl)  [unwired: 20 in, 3 out]
        n601 = control-ref of="FLUSHING FLOW RATE"() -> (w1776:refnum<vi>)
        n602 = call "PADMINI_AUTO_CYCLE_BIT3.vi"("Enum"=enum16{"Read", "Write"}."Read", "error in (no error)"=w1757) -> ("Input 2"=w1795:u16[])  [unwired: 8 in, 1 out]
        n603 = call "PADMINI_AUTO_BARCODE_STRING3.vi"("Enum"=enum16{"Read", "Write"}."Read", "error in (no error)"=w1757) -> ()  [unwired: 8 in, 2 out]
        n604 = call "PADMINI_AUTO_COUNTER_TIME3.vi"("Enum"=enum16{"Read", "Write"}."Read", "error in (no error)"=w1757) -> ("Input 2"=w1801:u16[])  [unwired: 8 in, 1 out]
        n605 = control-ref of="FLUSHING PRESSURE"() -> (w1775:refnum<vi>)
        n606 = call "PADMINI_BOOL_COLOR_CHANGE.vi"("error in (no error)"=w1757, "Numeric"=w1769, "Boolean in"=w1776) -> ("error out"=w1762:errorcluster)  [unwired: 8 in]
        n607 = Index Array(array=w1801) -> (element #1=w1778:u16, element #2=w1800:u16, element #3=w1799:u16, element #4=w1798:u16)  [unwired: 4 in]
        n608 = Index Array(array=w1795) -> (element=w1794:u16)  [unwired: 1 in]
        n609 = control-ref of="CALIBRATION LOAD VALUE"() -> (w1774:refnum<vi>)
        n610 = control-ref of="CALIBRATION DISPLACEMENT VALUE"() -> (w1773:refnum<vi>)
        n611 = control-ref of="CALIBRATION FLOW RATE"() -> (w1772:refnum<vi>)
        n612 = control-ref of="CALIBRATION PRESSURE"() -> (w1771:refnum<vi>)
        n613 = control-ref of="FIXING RING DISPLACEMENT"() -> (w1770:refnum<vi>)
        n614 = call "PADMINI_BOOL_COLOR_CHANGE.vi"("error in (no error)"=w1762, "Numeric"=w1768, "Boolean in"=w1775) -> ("error out"=w1761:errorcluster)  [unwired: 8 in]
        n615 = Divide(x=w1778, y=10.0) -> (x/y=w1777:dbl)
        n616 = Index Array(array=w1792, index=w1794) -> (element=w1793:string)
        n617 = call "PADMINI_BOOL_COLOR_CHANGE.vi"("error in (no error)"=w1761, "Numeric"=w1767, "Boolean in"=w1774) -> ("error out"=w1760:errorcluster)  [unwired: 8 in]
        n618 = call "PADMINI_BOOL_COLOR_CHANGE.vi"("error in (no error)"=w1760, "Numeric"=w1766, "Boolean in"=w1773) -> ("error out"=w1759:errorcluster)  [unwired: 8 in]
        n619 = call "PADMINI_BOOL_COLOR_CHANGE.vi"("error in (no error)"=w1759, "Numeric"=w1765, "Boolean in"=w1772) -> ("error out"=w1758:errorcluster)  [unwired: 8 in]
        n620 = call "PADMINI_BOOL_COLOR_CHANGE.vi"("error in (no error)"=w1758, "Numeric"=w1764, "Boolean in"=w1771) -> ("error out"=w1756:errorcluster)  [unwired: 8 in]
        n621 = call "PADMINI_BOOL_COLOR_CHANGE.vi"("error in (no error)"=w1756, "Numeric"=w1763, "Boolean in"=w1770) -> ("error out"=w1755:errorcluster)  [unwired: 8 in]
        n622 = local read "OP 40"() -> (w1809:T7)
        n623 = Bundle By Name(cluster=w1809, "STATUS"=w1793, "Cycle Time"=w1777, "OK Part"=w1800, "NOK Part"=w1799, "Total"=w1798, "Flushing Flow (Lph)"=w1789, "Flushing Pressure (Bar)"=w1788, "Calibration Load (KgF)"=w1754, "Calibration Displacement (mm)"=w1787, "Calibration Flow Rate (Lph)"=w1786, "Calibration Pressure (Bar)"=w1785, "Fixing Ring Displacement (mm)"=w1784, "PARAMETER 8"=w1783, "PARAMETER 9"=w1782, "PARAMETER 10"=w1781) -> (→"OP 40":T7)
        n624 = call "PADMINI_AUTO_CYCLE STATE3.vi"("Enum"=enum16{"Read", "Write"}."Read", "error in (no error)"=w1755) -> ("error out"=w1791:errorcluster, "Input 2"=w1805:u16[])  [unwired: 8 in]
        n625 = control-ref of="Cycle Status"() -> (w1751:refnum<vi>)
        n626 = control-ref of="Cycle Result"() -> (w1752:refnum<vi>)
        n627 = Index Array(array=w1805, index #1=0 ("index")) -> (element #1=w1804:u16, element #3=w1753:u16)  [unwired: 2 in, 1 out]
        n628 = call "PADMINI_STATUS_COLOR_CHANGE .vi"("Numeric"=w1804, "Boolean in"=w1751) -> ()  [unwired: 10 in]
        n629 = call "PADMINI_RESULT_COLOR_CHANGE .vi"("Numeric"=w1753, "Boolean in"=w1752) -> ()  [unwired: 10 in]
      }
      frame #3 {
        w1850 = 1.0 ("element")
        n630 = property on="OP 61" class="Clust"(error in=w1811) -> (error out=w1836:errorcluster, "Controls[]"=w1834:refnum<vi>[])  [unwired: 1 in, 1 out]
        n631 = property on="OP 60" class="Clust"(error in=w1811) -> (error out=w1843:errorcluster, "Controls[]"=w1861:refnum<vi>[])  [unwired: 1 in, 1 out]
        n632 = call "PADMINI_AUTO_CYCLE_BIT4.vi"("Enum"=enum16{"Read", "Write"}."Read", "error in (no error)"=w1811) -> ("Input 2"=w1882:u16[])  [unwired: 8 in, 1 out]
        n633 = call "PADMINI_AUTO_BARCODE_STRING4.vi"("Enum"=enum16{"Read", "Write"}."Read", "error in (no error)"=w1811) -> ()  [unwired: 8 in, 2 out]
        n634 = call "PADMINI_AUTO_COUNTER_TIME4.vi"("Enum"=enum16{"Read", "Write"}."Read", "error in (no error)"=w1811) -> ("Input 2"=w1875:u16[])  [unwired: 8 in, 1 out]
        n635 = call <vilib>:"Clear Errors.vi"("error in (no error)"=w1811) -> ("error out"=w1810:errorcluster)  [unwired: 5 in, 1 out]
        n636 = call "PADMINI_AUTO_RESULT_DATA_st4_log.vi"("Enum"=enum16{"Read", "Write"}."Read", "error in (no error)"=w1810) -> ("Input 2"=w1828:dbl[])  [unwired: 8 in, 1 out]
        n637 = call "PADMINI_AUTO_RESULT_DATA4.vi"("Enum"=enum16{"Read", "Write"}."Read", "error in (no error)"=w1811) -> ("Input 2"=w1867:dbl[])  [unwired: 8 in, 1 out]
        n638 = Index Array(array=w1875) -> (element #1=w1876:u16, element #2=w1877:u16, element #3=w1878:u16, element #4=w1879:u16)  [unwired: 4 in]
        n639 = Index Array(array=w1882) -> (element=w1883:u16)  [unwired: 1 in]
        n640 = Index Array(array=w1867) -> (element #1=w1868:dbl, element #2=w1849:dbl, element #3=w1859:dbl, element #4=w1848:dbl, element #5=w1858:dbl, element #6=w1857:dbl, element #7=w1856:dbl, element #8=w1855:dbl, element #9=w1854:dbl, element #10=w1853:dbl, element #11=w1817:dbl, element #12=w1852:dbl, element #13=w1851:dbl)  [unwired: 13 in]
        n641 = Array Subset(array=w1834, index=15, length=3) -> (w1833:refnum<vi>[])
        n642 = Index Array(array=w1828) -> (element #1=w1827:dbl, element #2=w1826:dbl, element #3=w1825:dbl, element #4=w1824:dbl, element #5=w1823:dbl, element #6=w1822:dbl, element #7=w1821:dbl)  [unwired: 8 in, 1 out]
        n643 = Array Subset(array=w1861, index=15, length=10) -> (w1862:refnum<vi>[])
        n644 = Index Array(array=w1885, index=w1883) -> (element=w1884:string)
        n645 = for {
          shift-right: [w1900] -> w1837
          shift-left: w1836 -> [w1900]
          tunnel: w1833 -> [w1902] mode=indexing
          tunnel: [w1899] -> w1835 mode=indexing
          w1901 = refnum<vi> refnum  # Boolean
          n646 = To More Specific Class(target class=w1901, reference=w1902) -> (specific class reference=w1899:refnum<vi>)  [unwired: 1 in, 1 out]
        }
        n647 = for {
          shift-right: [w1908] -> w1842
          shift-left: w1843 -> [w1908]
          tunnel: w1862 -> [w1910] mode=indexing
          tunnel: [w1907] -> w1845 mode=indexing
          w1909 = refnum<vi> refnum  # Boolean
          n648 = To More Specific Class(target class=w1909, reference=w1910) -> (specific class reference=w1907:refnum<vi>)  [unwired: 1 in, 1 out]
        }
        n649 = Build Array(w1823, w1822, w1821) -> (w1820:dbl[])
        n650 = Divide(x=w1876, y=u16 10) -> (x/y=w1819:dbl)
        n651 = local read "OP 61"() -> (w1839:T1)
        n652 = Build Array(w1817, w1852, w1851, w1850, w1850, w1850, w1850, w1850, w1850, w1850) -> (w1869:dbl[])
        n653 = for {
          tunnel: w1835 -> [w1898] mode=indexing
          tunnel: w1820 -> [w1897] mode=indexing
          tunnel: w1837 -> [w1896]
          tunnel: [w1895] -> w1838
          n654 = call "PADMINI_BOOL_COLOR_CHANGE.vi"("error in (no error)"=w1896, "Numeric"=w1897, "Boolean in"=w1898) -> ("error out"=w1895:errorcluster)  [unwired: 8 in]
        }
        n655 = for {
          tunnel: w1845 -> [w1906] mode=indexing
          tunnel: w1869 -> [w1905] mode=indexing
          tunnel: w1842 -> [w1904]
          tunnel: [w1903] -> w1841
          n656 = call "PADMINI_BOOL_COLOR_CHANGE.vi"("error in (no error)"=w1904, "Numeric"=w1905, "Boolean in"=w1906) -> ("error out"=w1903:errorcluster)  [unwired: 8 in]
        }
        n657 = Equal?(x=w1817, y=1.0) -> (x = y?=w1815:bool)
        n658 = disable-structure shown="Enabled" {
          disable-tunnel: w1838 -> [w1893 w1894]
          disable-tunnel: [w1887 w1894] -> w1830
          frame Disabled {
            n659 = call "PADMINI_AUTO_CYCLE STATE4.vi"("Enum"=enum16{"Read", "Write"}."Read", "error in (no error)"=w1893) -> ("error out"=w1887:errorcluster, "Input 2"=w1891:u16[])  [unwired: 8 in]
            n660 = control-ref of="Cycle Result"() -> (w1889:refnum<vi>)
            n661 = Index Array(array=w1891, index #1=0 ("index")) -> (element #3=w1888:u16)  [unwired: 2 in, 2 out]
            n662 = call "PADMINI_RESULT_COLOR_CHANGE .vi"("Numeric"=w1888, "Boolean in"=w1889) -> ()  [unwired: 10 in]
          }
          frame Enabled {
          }
        }
        "error out 3" <- w1830
        n663 = Select(t=TRUE, s=w1815, f=FALSE) -> (s? t:f=w1812:bool)
        n664 = Bundle By Name(cluster=w1839, "Pressure (Bar)"=w1827, "Actual Flow (Lpm)"=w1826, "lt Pressure (Bar)"=w1825, "Actual Flow (ccm)"=w1824) -> (→"OP 61":T1)
        n665 = call "PADMINI_AUTO_CYCLE STATE4.vi"("Enum"=enum16{"Read", "Write"}."Read", "error in (no error)"=w1841) -> ("error out"=w1886:errorcluster, "Input 2"=w1871:u16[])  [unwired: 8 in]
        n666 = global write "Global 1.vi" "STATION 2 OK"(w1812) -> ()
        n667 = local read "OP 60"() -> (w1863:T8)
        n668 = Bundle By Name(cluster=w1863, "STATUS"=w1884, "Cycle Time"=w1819, "OK Part"=w1877, "NOK Part"=w1878, "Total"=w1879, "Actual Flow (Lpm)"=w1868, "Pressure (Bar)"=w1849, "Actual Flow (ccm)"=w1859, "Pressure (Bar)"=w1848, "PARAMETER 5"=w1858, "PARAMETER 6"=w1857, "PARAMETER 7"=w1856, "PARAMETER 8"=w1855, "PARAMETER 9"=w1854, "PARAMETER 10"=w1853) -> (→"OP 60":T8)
        n669 = control-ref of="Cycle Status"() -> (w1844:refnum<vi>)
        n670 = control-ref of="Cycle Result"() -> (w1846:refnum<vi>)
        n671 = Index Array(array=w1871, index #1=0 ("index")) -> (element #1=w1872:u16, element #3=w1847:u16)  [unwired: 2 in, 1 out]
        n672 = call "PADMINI_STATUS_COLOR_CHANGE .vi"("Numeric"=w1872, "Boolean in"=w1844) -> ()  [unwired: 10 in]
        n673 = call "PADMINI_RESULT_COLOR_CHANGE .vi"("Numeric"=w1847, "Boolean in"=w1846) -> ()  [unwired: 10 in]
      }
    }
    n674 = local read "stop"() -> (w1595:bool)
    n675 = disable-structure shown="Enabled" {
      disable-tunnel: [u32 1000 ("milliseconds to wait") u32 100 ("milliseconds to wait")] -> w1585
      frame Disabled {
      }
      frame Enabled {
      }
    }
    n676 = Wait (ms)(milliseconds to wait=w1585) -> ()  [unwired: 1 out]
  }
  n677 = Release Queue(queue=w96, error in (no error)=w102) -> (error out=w75:errorcluster)  [unwired: 1 in, 2 out]
  n678 = call <vilib>:"Clear Errors.vi"("error in (no error)"=w98) -> ("error out"=w79:errorcluster)  [unwired: 5 in, 1 out]
  n679 = call <vilib>:"DB Tools Close Connection.vi"("error in (no error)"=w79, "connection reference"=w97) -> ("error out"=w76:errorcluster)  [unwired: 5 in]
  n680 = Merge Errors(w75, w76, w44) -> (w77:errorcluster)
  n681 = call <vilib>:"Simple Error Handler.vi"("error in (no error)"=w77) -> ("error out"=w72:errorcluster)  [unwired: 4 in, 4 out]
  n682 = call <vilib>:"Clear Errors.vi"("error in (no error)"=w72) -> ("error out"=w78:errorcluster)  [unwired: 5 in, 1 out]
  n683 = flat-sequence {
    tunnel: w78 -> [w1912]
    tunnel: [w1912] -> w80
    frame #0 {
      n684 = global write "Global 1.vi" "REMOVE VI"(TRUE ("remove_VI")) -> ()
    }
  }
  n685 = property class="App"(error in=w80) -> (error out=w82:errorcluster, "App.Kind"=w81:T10)  [unwired: 1 in, 1 out]
  n686 = case shown="\"Development System\", Default" w81 {
    tunnel: [w1913 w1915] -> w83
    tunnel: w82 -> [w1913 w1914]
    frame "Development System", Default {
    }
    frame "Run Time System" {
      n687 = invoke class="VI" method="FP.Close"(error in=w1914) -> (error out=w1915:errorcluster)  [unwired: 2 in, 2 out]
    }
  }
  "error out 2" <- w83
